vi "Dashboard Main.vi"() -> ()   [LabVIEW 2019]
uses:
  <vilib>/Utility/miscctls.llb/LVRectTypeDef.ctl
  <vilib>/Utility/miscctls.llb/LVRowAndColumnTypeDef.ctl
  <vilib>/event_ctls.llb/eventvkey.ctl
  <vilib>/Rock Robotics/WPI/DriverStation/WPI_DriverStationAllianceInfo.ctl
  <vilib>/Utility/xml.llb/Read From XML File(array).vi
  <vilib>/Utility/xml.llb/Write to XML File(string).vi
  <vilib>/Rock Robotics/Network Tables/NT Write Boolean.vi
  <vilib>/Rock Robotics/Network Tables/NT Read Boolean.vi
  <vilib>/Rock Robotics/Network Tables/NT Read Boolean Array.vi
  <vilib>/Rock Robotics/Network Tables/NT Write Boolean Array.vi
  <vilib>/Rock Robotics/WPI/Dashboard/WPI_DashboardLogging Global.vi
  <vilib>/vision/NI_Vision_Development_Module.lvlib
panel:
  out "Shifter_Faults_Array":bool[](array[boolean])
  out "Drive_Overheat_Array":bool[](array[boolean])
  out "Audible_Warnings_Enabled":bool
  in  "TCP":refnum<k5>
  in  "Rec Mode":enum32{"Stop", "Record", "Playback"}(radio)
  out "Image Message":string="Timeout in Camera Communications"
  in  "Dashboard Tab":T1(tab)=enum."Setup/Auto"
  in  "CheckList":i32(listbox)
  out "Match_End":bool
  out "Auto Playbook Entry":string
  out "Drive Action":string
  out "Subsystem Action":string
  in  "Driver Profile":u16(ring) items=["N/A"]
  in  "Camera Name":string(combo)="limelight"
  in  "Camera Settings":T2={"Frame Rate"=20, "Compression"=60, "Size"=1, "DB Camera Config"=FALSE} {"Size" items=["640x480", "320x240", "160x120"]}
  in  "Autonomous Play":u16(ring) items=["N/A"]
  out "Robot Pose":cluster{dbl[], dbl[]}[](graph)
  out "Master_Caution_0":bool caption="Mode_Butterfly"
  out "Robot_is_Autonomous_0":bool caption="Mode_Butterfly"
  in  "Robot Profile":u16(ring) items=["N/A"]
  out "Robot_Code_Version":string
  in  "Hide_Popups":bool
  in  "Default Camera Pipeline":u16(ring) items=["N/A"]
  in  "Dock_Dashboard":bool
  out "Auto_Suffix":string
  in  "Refresh_Auto_Play_List":bool
  in  "Force_Human_Control":bool
  in  "Auto_Test_Mode":bool
  in  "Auto_Delay":dbl format="%.1f"
  in  "Warning Time (s)":dbl=30.0 format="%.1f"
  in  "Manual_Start_X":dbl=509.25 format="%.1f"
  in  "Disable_Fusion_X":bool=TRUE
  out "Robot X":dbl format="%.1f"
  out "Robot Y":dbl format="%.1f"
  in  "Manual_Start_Y":dbl=94.66 format="%.1f"
  in  "Disable_Fusion_Y":bool=TRUE
  out "Robot H":dbl format="%.1f"
  in  "Manual_Start_H":dbl format="%.1f"
  out "Turret_H":dbl format="%.1f"
  out "Distance_To_Target_Detail":dbl format="%.1f"
  in  "Field Map":u16(ring) items=["N/A"]
  in  "Push_Robot_Start":bool
  in  "Export_Robot_Pose":bool
  in  "Clear_Robot_Pose_Display":bool
  in  "Driver_Help":bool
  in  "Error_Help":bool
  out "Help Graphic":T3(plugin-control)
  out "Drive_Train_Azimuth_Sensor":bool
  out "Camera_Fault":bool
  out "Robot Pose 1":cluster{dbl[], dbl[]}[](graph)
  out "Drive_Train_Shifter":bool
  out "Electrical_Fault":bool
  out "Diverting_Power":bool
  in  "Master_Safety_Override_1":bool
  out "Cowl_A":bool
  out "Cowl_B":bool
  out "Cowl_C":bool
  out "Shooter_Power":dbl(knob) scale=0.0..1.0
  out "Kicker_Power":dbl(knob) scale=0.0..1.0
  out "CAN_Bus_Fault":bool
  out "IMU_Failure":bool
  out "Robot_is_Autonomous_1":bool caption="Mode_Butterfly"
  in  "Pre_Spin":bool
  out "LL_Valid":bool caption="Mode_Butterfly"
  in  "Clear_Jams":bool
  out "Balls_Shot":i32 format="%#.0f"
  out "Ret_Feeder_Left":bool
  out "Ret_Feeder_Right":bool
  out "Climber_Climbing":bool caption="Mode_Butterfly"
  out "Tablet_Override":bool
  out "Match Time(s)":sgl format="%#.0f"
  out "Turret_Azimuth_Failure":bool
  out "Intake_Overheat":bool
  out "Flapper_Flapping":bool caption="Mode_Butterfly"
  out "Ret_Ball_Left":bool
  out "Ret_Ball_Right":bool
  in  "Emergency_Cowl_Retract":bool
  out "Shooter_Motor_Failure":bool
  out "Intake_On":bool caption="Mode_Butterfly"
  out "Shooter_Overheat":bool
  out "Ready_To_Shoot":bool caption="Mode_Butterfly"
  out "Auto_Error":bool
  in  "Clear_Errors":bool
  out "Drive_Train_Azimuth":bool
  out "Pressure_Transducer":dbl(slide) scale=0.0..120.0
  out "Pressure_Leak":bool
  out "Shooter_RPM_Actual":dbl(slide) scale=0.0..5700.0
  out "Drive_Train_Overheat":bool
  out "Compressor_On":bool
  out "Ret_Power_Port_Right":bool
  out "Ret_Power_Port_Left":bool
  in  "Right":bool
  in  "Reticule":T4(ring)
  in  "Save":bool
  in  "Up":bool
  in  "Down":bool
  in  "Left":bool
  out "Master_Caution_1":bool caption="Mode_Butterfly"
  out "Battery_Critical":bool
  out "Battery_Voltage":dbl(slide) scale=11.0..13.0
  out "Field_Oriented":bool caption="Mode_Butterfly"
  in  "Master_Safety_Override_2":bool
  out "Shooter_RPM_Goal":dbl(slide) scale=0.0..5700.0
  out "Slow_Loop":bool
  in  "Mode_TargetingComputer":bool
  in  "Mode_Wall":bool
  in  "Arm_Climber":bool
  in  "State_Normal":bool
  in  "State_Rotation_Control":bool
  in  "State_Climb":bool
  in  "Mode_InitiationLine":bool
  in  "Mode_CloseTrench":bool
  in  "Mode_FarTrench":bool
  in  "State_Position_Control":bool
  out "Combined Camera Feed":T3(plugin-control)
  out "High_Gear_0":bool
  out "High_Gear_1":bool
  out "High_Gear_2":bool
  out "High_Gear_3":bool
  in  "Camera_Override":bool
  out "Shooter_1_Temp":dbl
  out "Shooter_RPM_Goal_Detail":dbl
  out "Wheel_3S_Velocity":dbl format="%.1f"
  out "Wheel_3_Azimuth":dbl format="%.1f"
  out "Wheel_3S_Temp":dbl
  out "Wheel_0S_Temp":dbl
  in  "Select Auto":string(combo)="Select Autonomous ..."
  out "Camera Perf":string
  out "Control Loop Time (ms)":u32
  in  "Super_Test_Mode":bool
  in  "Calibrate_Wheels":bool
  in  "Zero_Wheels":bool
  out "Wheel_0_Azimuth":dbl format="%.1f"
  out "Wheel_0S_Velocity":dbl format="%.1f"
  out "Wheel_1S_Velocity":dbl format="%.1f"
  out "Wheel_1_Azimuth":dbl format="%.1f"
  out "Wheel_1S_Temp":dbl
  out "Wheel_2S_Velocity":dbl format="%.1f"
  out "Wheel_2_Azimuth":dbl format="%.1f"
  out "Wheel_2S_Temp":dbl
  in  "Arm_Calibrate":bool
  out "Shooter_0_RPM_Actual_Detail":dbl
  out "Master_Caution_2":bool caption="Mode_Butterfly"
  out "Shooter_0_Temp":dbl
  out "Shooter_1_RPM_Actual_Detail":dbl
  out "Out_Of_Range":bool
  in  "Wall_Speed":dbl=3000.0 min=0.0 max=5700.0 step=100.0
  in  "Initiation_Line":dbl=2250.0 min=0.0 max=5700.0 step=100.0
  in  "Close_Trench_Speed":dbl=2075.0 min=0.0 max=5700.0 step=100.0
  in  "Far_Trench_Speed":dbl=1975.0 min=0.0 max=5700.0 step=100.0
  out "Kicker_RPM_Actual_Detail":dbl
  out "Kicker_RPM_Goal_Detail":dbl
  out "Kicker_Temp":dbl
  in  "All_Kicker_Speed":dbl=4000.0 min=0.0 max=5700.0 step=100.0
  out "Intake_Temp":dbl
  out "Turret_Azimuth":dbl format="%.1f"
  in  "Arm_Calibrate_Turret":bool
  in  "Calibrate_Turret":bool
  in  "Turret_Override":bool
  in  "Actuator Testing":u16(ring) items=["N/A"]
  in  "Test_Actuator_Value":dbl step=0.1 format="%.2f"
  in  "Zero_Turret":bool
  in  "Auto_Target_Override":bool
  out "Turret_Limit_Switch_A":bool
  out "Turret_Limit_Switch_B":bool
  in  "Calibrate_Joysticks":bool
  in  "Arm_Calibrate_Joysticks":bool
  out "Robot_is_Autonomous_2":bool caption="Mode_Butterfly"
  in  "Test_Actuator_Period":dbl min=0.0 step=1.0 format="%.2f"
  out "Pose Loop Time (ms)":u32
  in  "Mute_Audible_Warnings":bool
  out "Combined Error String":string
  out "LIDAR_Distance_To_Target":dbl format="%.1f"
  out "Beam_Break_Raw":i32
  out "Wheel_0_Shifter_State":string
  out "Wheel_1_Shifter_State":string
  out "Wheel_3_Shifter_State":string
  out "Wheel_2_Shifter_State":string
  out "Azimuth_Error_Array":bool[](array[boolean])
  out "NT Connection":bool
  out "Mode":T5(ring)=enum."Auto Disabled"
  in  "Test Slider":dbl(slide) scale=0.0..100.0 scale format="%#_3g"
  in  "On/Off":bool caption="Solenoid"
  in  "Test Name":u16(ring) items=["Select the test to run..."]
  in  "Test Tree":string(tree)
  in  "Motor":cluster{"Value":dbl, "Enable":bool} {"Value" scale=-1.0..1.0 scale format="%#_3g"}
  out "Progress":T6 {"Test Progress" scale=0.0..100.0}
  in  "Rev/Fwd":cluster{"Forward":bool, "Reverse":bool}
  in  "Test Ring":u16(ring) items=["Monochrome", "Color"]
  out "Cmd Status":string
  in  "Execute Command":bool
  in  "Command Params":string[][](table)
  in  "Command Selection":i32(listbox)
  out "Tree":string(tree)
  out "Background":bool
  # "2020 Dashboard v3.5-stable"
  # "Auto Delay (s)"
  # "Auto Play Suffix"
  # "Robot X (in)"
  # "Endgame Alert (s)"
  # "Robot Y (in)"
  # "Robot H (deg)"
  # "Turret H (deg)"
  # "Undock Dashboard"
  # "Hide\nPopups"
  # "Auto Test\nMode"
  # "Force\nHuman"
  # "Distance (in)"
  # "Drive Action"
  # "Dock Dashboard"
  # "Dynamic Popups"
  # "Auto Real Mode"
  # "Robot\nDecides"
  # "Subsystem Action"
  # "11V"
  # "13V"
  # "0psi"
  # "120psi"
  # "High Gears"
  # "Shooter & Kicker"
  # "Miscellaneous"
  # "Drive Train"
  # "Calibrate Joysticks"
  # "Control"
  # "Pose"
  # "LIDAR\nDistance (in)"
  # "Latency\n(ms)"
  # "Intake"
  # "Module 1"
  # "Module 0"
  # "Shooter"
  # "Kicker"
  # "Azimuth (deg)"
  # "Temp (C)"
  # "Speed Goal (rpm)"
  # "Temp (C)"
  # "Beam Break"
  # "Turret \nOverride"
  # "Auto Target Override"
  # "Camera Override"
  # "Super Test Mode"
  # "Shoot 0"
  # "Shoot 1"
  # "Kicker"
  # "Turret"
  # "Velocity (ft/s)"
  # "Speed (rpm)"
  # "Azimuth (deg)"
  # "Shifter State"
  # "Temp (C)"
  # "Limits"
  # "Module 2"
  # "Module 3"
  # "Setpoints (not saved)"
  # "Azimuth (deg)"
  # "Normal\nTurret"
  # "Normal \nAuto Target"
  # "Normal Camera"
  # "Safe"
  # "Close \nWall"
  # "Initiation\nLine"
  # "Close\nTrench"
  # "Mid\nTrench"
  # "All \nKicker"
  # "Calibrate Turret"
  # "Temp (C)"
  # "Velocity (ft/s)"
  # "(rpm)"
  # "Shifter State"
  # "p: power [-1,1]\nb: boolean {0,1}\nRPM: speed\na: angle [0,+inf)"
  # "Amplitude"
  # "Calibrate Wheels"
  # "Period (s)"
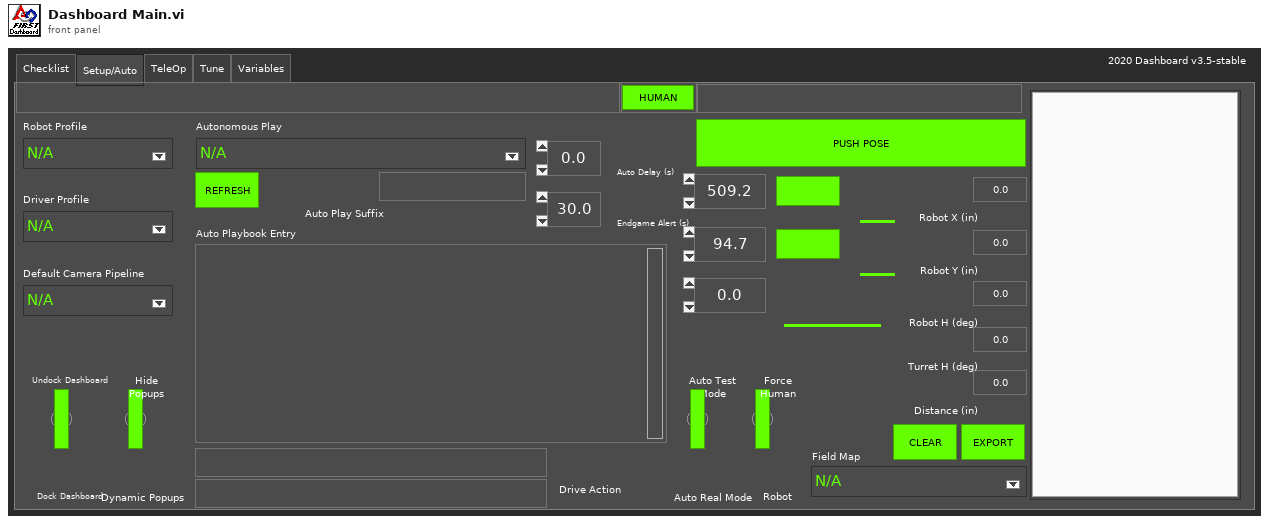
[diagram p1: front panel]
types:
  T1 = enum32{"Checklist", "Setup/Auto", "TeleOp", "Tune", "NT", "Test", "Commands", "Variables"}
  T2 = cluster{"Frame Rate":i32, "Compression":i32, "Size":u16, "DB Camera Config":bool}
  T3 = typedef "IMAQ Image.ctl" = refnum<image>
  T4 = enum16{"Power Port Left", "Power Port Right", "Ball Left", "Ball Right", "Feeder Left", "Feeder Right"}
  T5 = enum8{"Tele-Op Disabled", "Tele-Op Enabled", "Auto Disabled", "Auto Enabled", "Test Disabled", "Test Enabled", "Disconnected", "No Code", "E-Stop"}
  T6 = cluster{"Test Progress":u8, "Test Progress Text":string}
  T7 = cluster{"Save Path":path, "Interval (s)":dbl, "Keep":i32}
  T8 = enum32{"Drive", "Camera", "Basic", "Custom", "Test", "Commands", "Checklist", "Variables"}
  T9 = cluster{"IDs":cluster{"RPC field ID":u16, "Unique ID":u16}, "String":string}
  T10 = typedef "Image Type" = u32
  T11 = cluster{"Ret_Power_Port_Left":refnum<vi>, "Ret_Power_Port_Right":refnum<vi>, "Ret_Ball_Left":refnum<vi>, "Ret_Ball_Right":refnum<vi>, "Ret_Feeder_Left":refnum<vi>, "Ret_Feeder_Right":refnum<vi>}
  T12 = cluster{"Camera Name":string, string, "Saved DB Images Info":cluster{"Save Path":path, "Interval (s)":dbl, "Keep":i32}}
  T13 = enum8{"Enabled", "Disabled", "Disabled and Grayed Out"}
  T14 = typedef "WPI_DriverStationAllianceInfo.ctl" = enum16{"Red", "Blue", "Invalid"}
  T15 = cluster{"Error Strings":string, "Disable Counts":cluster{u16, u16}, "Rail Faults":cluster{u16, u16, u16}, "Robot IP":string, "DB Mode":u8, "Event Info":cluster{"Name":string, "Type":u8, "Number":u16, "Replay":u8}}
  T16 = cluster{"Storage":cluster{"Disk Free":u64, "RAM Block":u32, "RAM free":u32}, "CPU Utilization":cluster{"CPU % ISR":sgl, "CPU % Time Crit":sgl, "CPU % Timed Str":sgl, "CPU % High":sgl, "CPU % Above":sgl, "CPU % Normal":sgl, "CPU % Low":sgl}, "CAN":cluster{"% Bus Utilization":sgl, "Bus Off Cnt":u32, "TX_FIFO Full Cnt":u32, "Receive Error Cnt":u8, "Transmit Error Cnt":u8}, "HID":cluster{"HID Outputs":u32, "Rumble Low":u16, "Rumble High":u16}[]}
  T17 = cluster{"Status bits":cluster{"Test Mode":bool, "Autonomous":bool, "Enabled":bool, "Code Start":bool, "Brownout":bool, "Reserved 2":bool, "Reserved 3":bool, "E-Stop":bool}, "Code Trace":cluster{"Disabled":bool, "TeleOp":bool, "Auto":bool, "Test":bool}, "Controller Type":enum16{"unknown", "cRIO", "roboRio"}, "Code?":enum16{"unknown", "noCode", "code"}, "Battery V":dbl}
  T18 = cluster{"Control Bits":cluster{"TestMode":bool, "Autonomous":bool, "Enabled":bool, "FMS Present":bool, bool, bool, bool, "E-Stop":bool}, "Team Station ":u8, "Countdown":sgl, "Joystick Values":cluster{"Axes":dbl[], "Buttons":bool[], "POVs":i16[]}[]}
  T19 = typedef "imagedata.ctl" = cluster{"image type":i32, "image depth":i32, "image":u8[], "mask":u8[], "colors":u32[], "Rectangle":cluster{"left":i16, "top":i16, "right":i16, "bottom":i16}}
  T20 = cluster{bool, "Super_Test_Mode":bool, "Slow_Loop":bool, "Drive_Train_Overheat":bool, "Pressure_Leak":bool, "Drive_Train_Azimuth":bool, "Arm_Calibrate":bool, "Auto_Error":bool, "Auto_Test_Mode":bool, "Shooter_Overheat":bool, "Shooter_Motor_Failure":bool, "Intake_Overheat":bool, "Turret_Azimuth_Failure":bool, "Arm_Calibrate_Turret":bool, bool, "IMU_Failure":bool, "Electrical_Fault":bool, "Arm_Calibrate_Joysticks":bool, "CAN_Bus_Fault":bool, "Drive_Train_Shifter":bool, "Drive_Train_Azimuth_Sensor":bool, "Battery_Critical":bool}
  T21 = cluster{"Operation":enum16{"Update", "Clear"}, "Color Box":u32}[]
  T22 = typedef "eventvkey.ctl" = enum16{"ASCII", "Enter", "Return", "Shift", "Ctrl", "Alt", "Cmd", "Opt", "Caps", "NumLock", "Clear", "Break", "Up", "Down", "Left", "Right", "Insert", "Delete", "Home", "End", "PageUp", "PageDown", "Escape", "Help", "Pause", "ScrollLock", "F1", "F2", "F3", "F4", "F5", "F6", "F7", "F8", "F9", "F10", "F11", "F12", "F13", "F14", "F15", "F16", "F17", "F18", "F19", "F20", "F21", "F22", "F23", "F24", "Play", "VolumeUp", "VolumeDown", "Mute", "Two Byte Char"}
  T23 = cluster{"Image Size":bool, "Image Type":bool, "Pixel Value":bool, "ROI Information":bool, "Zoom Factor":bool}
  T24 = cluster{"Operation":enum16{"Update", "Clear"}, "Color Box":u32}
  T25 = typedef "LVRowAndColumnTypeDef.ctl" = cluster{"Row":i32, "Column":i32}
  T26 = cluster{"Shift":bool, "Ctrl":bool, "Alt":bool, "Cmd":bool, "Opt":bool}
  T27 = cluster{string, "Drive_Train_Azimuth_Sensor":bool, dbl}
  T28 = cluster{string, "Drive_Train_Overheat":bool, dbl}
  T29 = cluster{string, "Shooter_Motor_Failure":bool, dbl}
  T30 = cluster{string, "Turret_Azimuth_Failure":bool, dbl}
  T31 = cluster{string, "Arm_Calibrate_Turret":bool, dbl}
  T32 = cluster{string, "Arm_Calibrate_Joysticks":bool, dbl}
  T33 = cluster{string, "Drive_Train_Azimuth_Sensor":bool, dbl}[]
  T34 = typedef "LVRectTypeDef.ctl" = cluster{"Left":i16, "Top":i16, "Right":i16, "Bottom":i16}
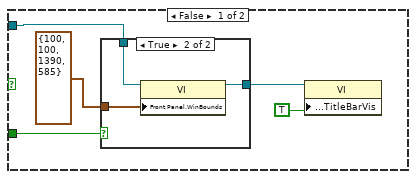
[diagram p2: hidden frame]
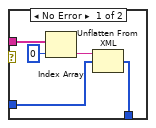
[diagram p6: hidden frame]
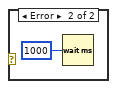
[diagram p9: hidden frame]
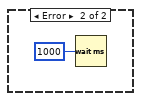
[diagram p10: hidden frame]
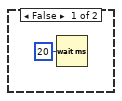
[diagram p11: hidden frame]
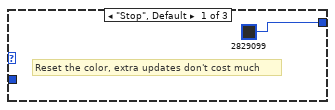
[diagram p15: hidden frame]
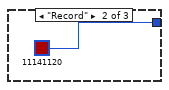
[diagram p16: hidden frame]
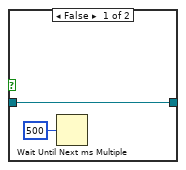
[diagram p19: hidden frame]
diagram:
  w5 = T7 {"Save Path"=path "", "Interval (s)"=1.0, "Keep"=180}  # Saved DB Images Info
  w4 = "Left"
  w16 = T9 {"IDs"={"RPC field ID"=0, "Unique ID"=0}, "String"=""}  # RPC Response
  w26 = enum32{"Stop", "Record", "Playback"}."Stop" ("Rec Mode")
  w20 = FALSE ("Visible")
  w42 = T10 4 items=["Grayscale (U8)", "Grayscale (I16)", "Grayscale (SGL)", "Complex (CSG)", "RGB (U32)", "HSL (U32)", "RGB (U64)"] ("Image Type")
  # "Started one, Unique ID holds\nresponse"
  # "Loop 7. Wait for DS connections"
  # "Basic debug and auto controls: Their data names are fixed, but\nthe displayed name, called a caption, can be changed directly or in\nrobot code such as shown in Begin."
  # "Controls for Test Mode, Camera Settings, etc."
  # "Additional UI Initialization"
  # "Loop 6. Animation for background of window during playback and record"
  # "Fires each time robot IP\nchanges, simulator does this"
  # "Fires each time window\ndocking changes."
  # "The remaining code below this line typically doesn't need to be modified."
  # "Loop 4. Process UI events related to test mode, checklist, and camera settings"
  # "Loop 3. Wait until the robot response provides\n the Robot IP address.\nOnce known, bind controls and\nvariables with the same names."
  n1 = control-ref of="Dashboard Tab"() -> (w24:refnum<vi>)
  n2 = control-ref of="Camera Name"() -> (w11:refnum<vi>)
  n3 = control-ref of="Camera Settings"() -> (w3:refnum<vi>)
  n4 = property class="VI" props=["Front Panel.Closeable"]() -> (reference out=w25:refnum<vi>)  [unwired: 2 in, 2 out]
  n5 = call <vilib>:"Get Tab Control Refs.vi"("Page Index"=T8."Basic" ("Dashboard Tab"), "TabControl in"=w24) -> ("ControlsOnPage"=w10:refnum<vi>[])  [unwired: 9 in]
  n6 = Obtain Notifier(name (unnamed)="Window Mode", notification data type=TRUE) -> (notifier out=w19:refnum<notifier>)  [unwired: 2 in, 2 out]
  n7 = call <vilib>:"Get Tab Control Refs.vi"("Page Index"=T8."Custom" ("Dashboard Tab"), "TabControl in"=w24) -> ("ControlsOnPage"=w23:refnum<vi>[])  [unwired: 9 in]
  n8 = Obtain Notifier(name (unnamed)="Robot IP Update", notification data type="IP Addr" ("name (unnamed)")) -> (notifier out=w2:refnum<notifier>)  [unwired: 2 in, 2 out]
  n9 = Create User Event(user event datatype=w16) -> (user event=w13:refnum<user-event>)  [unwired: 1 in, 1 out]
  n10 = call "IMAQ Create"("Image Name"="Full Video Stream", "Image Type"=w42) -> ("New Image"=w41:T3, "error out"=w40:errorcluster)  [unwired: 2 in, 1 out]
  n11 = Build Array (concatenate)(w10, w23) -> (w22:refnum<vi>[])
  n12 = control-ref of="CheckList"() -> (w21:refnum<vi>)
  n13 = call "Handle Camera Configuration.vi"("CameraNameRef"=w11, "Display Name"=w4, "ClusterRef"=w3) -> ()  [unwired: 9 in]
  n14 = register-events(refnum<vi> refnum, w13) -> (reference out=w30:refnum<event-registration>, error out=w29:errorcluster)  [unwired: 2 in]
  n15 = while {
    tunnel: w22 -> [w54]
    tunnel: w2 -> [w52]
    tunnel: [w50] -> _
    tunnel: u32 1000 ("milliseconds to wait") -> [w49]
    tunnel: w13 -> [w43]
    i -> [w50]
    stop <- FALSE stop-if-true
    n16 = local read "Rec Mode"() -> (w45:enum32{"Stop", "Record", "Playback"})
    n17 = Wait on Notification(notifier=w52, timeout in ms (-1)=w49) -> (notification=w51:string, timed out?=w47:bool)  [unwired: 2 in, 2 out]
    n18 = Equal?(x=w45, y=u16 2 ("Rec Mode")) -> (x = y?=w46:bool)
    n19 = Compound Arithmetic op=OR(invert w47, w46) -> (w48:bool)
    n20 = case shown="True" w48 {
      tunnel: w54 -> [_ w57]
      tunnel: w51 -> [_ w56]
      tunnel: w43 -> [_ w55]
      frame False {
      }
      frame True {
        n21 = call <vilib>:"Bind Controls to SmartDashboard.vi"("RPC ref"=w55, "Bound Control Refs"=w57, "Server IP Address"=w56) -> ()  [unwired: 9 in]
      }
    }
  }
  n22 = while {
    shift-right: [w76] -> _
    shift-left: _ -> [w129]
    shift-right: [w77] -> _
    shift-left: _ -> [w119]
    tunnel: w2 -> [_]
    stop <- FALSE stop-if-true
    # "Dynamic Overlays"
    n23 = To Long Integer(number="Reticule") -> (32bit integer=w110:i32)
    n24 = Wait (ms)(milliseconds to wait=u32 100) -> ()  [unwired: 1 out]
    n25 = Multiply(x=w110, y=2) -> (x*y=w109:i32)
    n26 = control-ref of="Ret_Power_Port_Left"() -> (w90:refnum<vi>)
    n27 = control-ref of="Ret_Power_Port_Right"() -> (w89:refnum<vi>)
    n28 = control-ref of="Ret_Ball_Left"() -> (w75:refnum<vi>)
    n29 = control-ref of="Ret_Ball_Right"() -> (w74:refnum<vi>)
    n30 = control-ref of="Ret_Feeder_Left"() -> (w63:refnum<vi>)
    n31 = control-ref of="Ret_Feeder_Right"() -> (w62:refnum<vi>)
    n32 = Increment(x=w109) -> (x+1=w96:i32)
    n33 = First Call?() -> (First Call?: T/F=w99:bool)
    n34 = Index Array(array=w119, index #1=w109, index #2=w96) -> (element #1=w113:i32, element #2=w121:i32)
    n35 = Or(x="Up", y="Down") -> (x .or. y?=w125:bool)
    n36 = Or(x="Left", y="Right") -> (x .or. y?=w115:bool)
    n37 = case shown="True" w99 {
      tunnel: [w140 w159] -> w76
      tunnel: w129 -> [w140 _]
      tunnel: w90 -> [_ w158]
      tunnel: w89 -> [_ w157]
      tunnel: w75 -> [_ w148]
      tunnel: w74 -> [_ w147]
      tunnel: w63 -> [_ w142]
      tunnel: w62 -> [_ w141]
      frame False {
      }
      frame True {
        n38 = property class="Bool (strict)"(reference=w158) -> ("Left"=w156:i32, "Top"=w155:i32)  [unwired: 1 in, 2 out]
        n39 = property class="Bool (strict)"(reference=w157) -> ("Left"=w154:i32, "Top"=w153:i32)  [unwired: 1 in, 2 out]
        n40 = property class="Bool (strict)"(reference=w148) -> ("Left"=w152:i32, "Top"=w151:i32)  [unwired: 1 in, 2 out]
        n41 = property class="Bool (strict)"(reference=w147) -> ("Left"=w150:i32, "Top"=w149:i32)  [unwired: 1 in, 2 out]
        n42 = property class="Bool (strict)"(reference=w142) -> ("Left"=w146:i32, "Top"=w145:i32)  [unwired: 1 in, 2 out]
        n43 = property class="Bool (strict)"(reference=w141) -> ("Left"=w144:i32, "Top"=w143:i32)  [unwired: 1 in, 2 out]
        n44 = Build Array(w156, w155, w154, w153, w152, w151, w150, w149, w146, w145, w144, w143) -> (w159:i32[])
      }
    }
    n45 = Bundle("Ret_Power_Port_Left"=w90, "Ret_Power_Port_Right"=w89, "Ret_Ball_Left"=w75, "Ret_Ball_Right"=w74, "Ret_Feeder_Left"=w63, "Ret_Feeder_Right"=w62) -> (w81:T11)  [unwired: 1 in]
    n46 = Decrement(x=w121) -> (x-1=w128:i32)
    n47 = Increment(x=w121) -> (x+1=w127:i32)
    n48 = Decrement(x=w113) -> (x-1=w118:i32)
    n49 = Increment(x=w113) -> (x+1=w117:i32)
    n50 = Select(t=w128, s="Up", f=w127) -> (s? t:f=w126:i32)
    n51 = Select(t=w118, s="Left", f=w117) -> (s? t:f=w116:i32)
    n52 = Select(t=w126, s=w125, f=w121) -> (s? t:f=w95:i32)
    n53 = Select(t=w116, s=w115, f=w113) -> (s? t:f=w114:i32)
    n54 = Replace Array Subset(array=w119, new element #1=w114, index #1=w109, new element #2=w95, index #2=w96) -> (w94:i32[])
    n55 = Current VI's Path() -> (path=w105:path)
    n56 = Strip Path(path=w105) -> (stripped path=w104:path)  [unwired: 1 out]
    n57 = Cluster To Array(cluster=w81) -> (array=w93:refnum<vi>[])
    n58 = Strip Path(path=w104) -> (stripped path=w103:path)  [unwired: 1 out]
    n59 = Array Size(array=w93) -> (size(s)=w92:i32)
    n60 = Build Path(base path=w103, name or relative path=path "reticule positions.txt" ("XML File Path")) -> (appended path=w102:path)
    n61 = Multiply(x=2 ("dimension size"), y=w92) -> (x*y=w98:i32)
    n62 = Initialize Array(0, w98) -> (w88:i32[])
    n63 = call-poly <vilib>:"Read From XML File.vi"("XML File Path"=w102) -> ("error out"=w80:errorcluster, "XML Elements"=w101:string[])  [unwired: 8 in, 1 out]
    n64 = case shown="Error .." w80 {
      tunnel: w101 -> [w136 _]
      tunnel: w88 -> [w133 _]
      tunnel: [w132 i32[] [0, 0, 0, 0, 0, 0, 0, 0, 0, 0, 0, 0] ("value")] -> w78
      frame No Error {
        n65 = Index Array(array=w136, index=0) -> (element=w134:string)
        n66 = Unflatten From XML(xml string=w134, type=w133) -> (value=w132:i32[])  [unwired: 1 in, 1 out]
      }
      frame Error {
      }
    }
    n67 = First Call?() -> (First Call?: T/F=w120:bool)
    n68 = Select(t=w78, s=w120, f=w94) -> (s? t:f=w77:i32[])
    n69 = Add(x=w77, y=w76) -> (x+y=w79:i32[])
    n70 = Index Array(array=w79, index #1=0 ("index")) -> (element #1=w85:i32, element #2=w84:i32, element #3=w83:i32, element #4=w82:i32, element #5=w73:i32, element #6=w72:i32, element #7=w71:i32, element #8=w70:i32, element #9=w67:i32, element #10=w66:i32, element #11=w65:i32, element #12=w64:i32)  [unwired: 11 in]
    n71 = Unbundle(w81) -> ("Ret_Power_Port_Left"=w86:refnum<vi>, "Ret_Power_Port_Right"=w87:refnum<vi>, "Ret_Ball_Left"=w69:refnum<vi>, "Ret_Ball_Right"=w68:refnum<vi>, "Ret_Feeder_Left"=w61:refnum<vi>, "Ret_Feeder_Right"=w60:refnum<vi>)
    n72 = Flatten To XML(anything=w77) -> (xml string=w107:string)
    n73 = call "EdgeTrigger.vi"("Input Signal"="Save") -> ("Rising Edge Trigger"=w58:bool)  [unwired: 2 out]
    n74 = case shown="True" w58 {
      tunnel: w107 -> [_ w139]
      tunnel: w102 -> [_ w138]
      frame False {
      }
      frame True {
        n75 = call-poly <vilib>:"Write to XML File.vi"("XML Input"=w139, "XML File Path"=w138) -> ()  [unwired: 7 in, 3 out]
      }
    }
    n76 = property class="Bool (strict)"(reference=w86, "Left"=w85, "Top"=w84) -> ()  [unwired: 1 in, 2 out]
    n77 = property class="Bool (strict)"(reference=w87, "Left"=w83, "Top"=w82) -> ()  [unwired: 1 in, 2 out]
    n78 = property class="Bool (strict)"(reference=w69, "Left"=w73, "Top"=w72) -> ()  [unwired: 1 in, 2 out]
    n79 = property class="Bool (strict)"(reference=w68, "Left"=w71, "Top"=w70) -> ()  [unwired: 1 in, 2 out]
    n80 = property class="Bool (strict)"(reference=w61, "Left"=w67, "Top"=w66) -> ()  [unwired: 1 in, 2 out]
    n81 = property class="Bool (strict)"(reference=w60, "Left"=w65, "Top"=w64) -> ()  [unwired: 1 in, 2 out]
  }
  n82 = while {
    tunnel: w41 -> [w175]
    tunnel: w40 -> [_]
    tunnel: w5 -> [w180]
    tunnel: w4 -> [w178]
    stop <- FALSE stop-if-true
    # "Camera Feeds"
    n83 = local read "NT Connection"() -> (w181:bool)
    n84 = local read "Rec Mode"() -> (w182:enum32{"Stop", "Record", "Playback"})
    n85 = Bundle("Camera Name"="Camera Name", w178, "Saved DB Images Info"=w180) -> (w179:T12)  [unwired: 1 in]
    n86 = control-ref of="Camera Perf"() -> (w176:refnum<vi>)
    n87 = call <vilib>:"WPI_CameraRead MJPG for Dashboard_2.vi"("Camera Settings"="Camera Settings", "Rec Mode"=w182, "NT Connection"=w181, "Capture Info"=w179, "Image in"=w175) -> ("perf info"=w177:cluster{"Bandwidth (Mbps)":dbl, "fps":dbl}, "Active"=w183:bool, "Image\\ out"=w184:T3)  [unwired: 4 in]
    n88 = call <vilib>:"WPI_DashboardFormatPerf.vi"("Right Camera Perf"=cluster{"Bandwidth (Mbps)":dbl, "FPS":dbl} {"Bandwidth (Mbps)"=0.0, "FPS"=0.0}, "Performance"=w177, "String in"=w176) -> ()  [unwired: 9 in]
    n89 = case shown="True" w183 {
      tunnel: w184 -> [w197 w200]
      tunnel: [w197 w199] -> w174
      frame False {
        n90 = Wait Until Next ms Multiple(millisecond multiple=u32 500) -> ()  [unwired: 1 out]
      }
      frame True {
        # "image annotation etc."
        n91 = call "IMAQ Clear Overlay"("Image"=w200) -> ("Image Out"=w199:T3)  [unwired: 2 in, 8 out]
      }
    }
    n92 = call "IMAQ Rotate"("Angle (degrees)"=sgl 0.0, "Image Src"=w174) -> ("Image Dst Out"=w163:T3)  [unwired: 8 in, 1 out]
    n93 = call "IMAQ GetImageSize"("Image"=w163) -> ("Y Resolution"=w169:i32, "X Resolution"=w170:i32)  [unwired: 3 in, 1 out]
    n94 = To Double Precision Float(number=w170) -> (double precision float=w172:dbl)
    n95 = To Double Precision Float(number=w169) -> (double precision float=w171:dbl)
    n96 = Divide(x=w172, y=w171) -> (x/y=w168:dbl)
    n97 = Less?(x=w168, y=1.5) -> (x < y?=w160:bool)
    "Camera_Fault" <- w160
    n98 = case shown="True" w160 {
      tunnel: "Partial Video Stream" ("Image Name") -> [_ w196]
      tunnel: [w186 w195] -> w162
      tunnel: w163 -> [w186 w191]
      frame False {
        # "wide angle camera found"
      }
      frame True {
        # "no wide angle camera found"
        n99 = call "IMAQ GetImageInfo"("Image"=w191) -> ("Y Resolution"=w190:i32, "X Resolution"=w189:i32, "Image Type"=w194:T10)  [unwired: 3 in, 5 out]
        n100 = call "IMAQ Create"("Image Name"=w196, "Image Type"=w194) -> ("New Image"=w193:T3)  [unwired: 3 in, 1 out]
        n101 = Multiply(x=w189, y=2) -> (x*y=w188:i32)
        n102 = call "IMAQ SetImageSize"("Y Resolution"=w190, "X Resolution"=w188, "Image"=w193) -> ("Image Out"=w192:T3)  [unwired: 2 in, 1 out]
        n103 = call "IMAQ ImageToImage 2"("Image Src (Small)"=w191, "Image Src (Large)"=w192) -> ("Image Dst Out"=w195:T3)  [unwired: 8 in, 1 out]
      }
    }
    "Combined Camera Feed" <- w162
  }
  n104 = call "Initialize Camera and CheckList.vi"("ListBox in"=w21) -> ()  [unwired: 11 in]
  n105 = control-ref of="Test Tree"() -> (w35:refnum<vi>)
  n106 = while {
    tunnel: w2 -> [w204]
    tunnel: w19 -> [w201]
    stop <- FALSE stop-if-true
    n107 = call <vilib>:"WPI_DashboardRetrieveStatusInfo.vi"("Binding Refnum"=w204, "Window Mode Notifier"=w201, "TCP Cnx"="TCP") -> ("Power and Errors"=w205:T15, "Robot Metrics"=w208:T16, "Status Info"=w209:T17, "Control Info"=w206:T18, "Robot Mode"=w203:T5, "Process?"=w207:bool)  [unwired: 3 in]
    "Mode" <- w203
    n108 = case shown="True" w207 {
      tunnel: w209 -> [_ _]
      tunnel: w208 -> [_ _]
      tunnel: w206 -> [_ _]
      tunnel: w205 -> [_ _]
      tunnel: w203 -> [_ _]
      frame False {
        n109 = Wait (ms)(milliseconds to wait=u32 20) -> ()  [unwired: 1 out]
      }
      frame True {
        w216 = "H" ("x")
        w222 = bool[] [FALSE, FALSE, FALSE, FALSE] ("Default Value")
        w269 = FALSE  # Compressor
        w264 = FALSE
        w272 = FALSE  # LimeLight
        w595 = cluster{u32, u32}[] [{15663313, 16448250}, {16448250, 16448250}] ("Un-selected Color")
        w541 = cluster{u32, u32}[] [{9567230, 16448250}, {16448250, 16448250}] ("Un-selected Color")
        # "# of false elements"
        # "Find # of trues"
        # "manage audible warnings"
        # "robot configuration"
        # "manipulator controls"
        # "spinner reporting"
        # "report targeting information"
        # "report tab position"
        # "tuning parameters and calibrations"
        # "climber reporting"
        # "turret reporting"
        # "intake and magazine reporting"
        # "drive system reporting"
        # "report resource usage"
        # "dynamic overlays"
        # "shooter reporting"
        # "shooter state controller"
        # "master state controller"
        # "report match time"
        # "actuator test interlocks"
        # "emergency overrides"
        # "caution alarms"
        # "driver configuration"
        # "autonomous reporting"
        # "autonomous configuration"
        # "display auto \nplaybook"
        n110 = call-poly <vilib>:"NT Read Value.vi"("Name"="Alliance_Color") -> ("Numeric"=w702:dbl)  [unwired: 9 in, 1 out]
        n111 = To Unsigned Word Integer(number=w702) -> (unsigned 16bit integer=w701:u16)
        n112 = call-poly <vilib>:"NT Read Value.vi"("Name"="Robot_Mode") -> ("String"=w343:string)  [unwired: 9 in, 1 out]
        n113 = Build Array("N/A") -> (w791:string[])
        n114 = call-poly <vilib>:"NT Read Value.vi"("Default Value"=0.0, "Name"="Robot_H") -> ("Numeric"=w351:dbl)  [unwired: 8 in, 1 out]
        n115 = call-poly <vilib>:"NT Read Value.vi"("Default Value"=0.0, "Name"="Turret_H") -> ("Numeric"=w350:dbl)  [unwired: 8 in, 1 out]
        n116 = feedback-in #1(w701) -> ()
        n117 = feedback #1(w701) -> (w709:u16)
        n118 = Not Equal?(x=w701, y=w709) -> (x != y?=w707:bool)
        n119 = feedback #2("Field Map") -> (w301:u16)
        n120 = feedback-in #2("Field Map") -> ()
        n121 = Not Equal?(x="Field Map", y=w301) -> (x != y?=w299:bool)
        n122 = call-poly <vilib>:"NT Read Value.vi"("Default Value"=-1.0, "Name"="Robot_Y") -> ("Numeric"=w353:dbl)  [unwired: 8 in, 1 out]
        "Robot Y" <- w353
        n123 = call-poly <vilib>:"NT Read Value.vi"("Default Value"=-1.0, "Name"="Robot_X") -> ("Numeric"=w354:dbl)  [unwired: 8 in, 1 out]
        "Robot X" <- w354
        n124 = First Call?() -> (First Call?: T/F=w708:bool)
        n125 = call-poly <vilib>:"NT Read Value.vi"("Default Value"=w791, "Name"="Legal_Auto_Plays") -> ("String Array"=w789:string[])  [unwired: 8 in, 1 out]
        n126 = To Double Precision Float(number="Autonomous Play") -> (double precision float=w795:dbl)
        n127 = call-poly <vilib>:"NT Read Value.vi"("Default Value"="Waiting for connection...", "Name"="Auto_Playbook") -> ("String"=→"Auto Playbook Entry":string)  [unwired: 8 in, 1 out]
        n128 = Quotient & Remainder(x=w351, y=360.0) -> (x-y*floor(x/y)=→"Robot H":dbl)  [unwired: 1 out]
        n129 = Quotient & Remainder(x=w350, y=360.0) -> (x-y*floor(x/y)=→"Turret_H":dbl)  [unwired: 1 out]
        n130 = call-poly <vilib>:"NT Read Value.vi"("Name"="Auto_Path_Suffix") -> ("String"=→"Auto_Suffix":string)  [unwired: 9 in, 1 out]
        n131 = Compound Arithmetic op=OR(w707, w708, w299) -> (w706:bool)
        n132 = call-poly <vilib>:"NT Write Value.vi"("Boolean"="Disable_Fusion_X", "Name"="Disable_Fusion_X") -> ()  [unwired: 9 in, 1 out]
        n133 = call-poly <vilib>:"NT Write Value.vi"("Boolean"="Disable_Fusion_Y", "Name"="Disable_Fusion_Y") -> ()  [unwired: 9 in, 1 out]
        n134 = call-poly <vilib>:"NT Write Value.vi"("Boolean"="Push_Robot_Start", "Name"="Push_Robot_Start") -> ()  [unwired: 9 in, 1 out]
        n135 = call-poly <vilib>:"NT Write Value.vi"("Boolean"="Auto_Test_Mode", "Name"="Auto_Test_Mode") -> ()  [unwired: 9 in, 1 out]
        n136 = call-poly <vilib>:"NT Write Value.vi"("Numeric"="Auto_Delay", "Name"="Auto_Delay") -> ()  [unwired: 9 in, 1 out]
        n137 = call-poly <vilib>:"NT Write Value.vi"("Numeric"="Manual_Start_X", "Name"="Manual_Start_X") -> ()  [unwired: 9 in, 1 out]
        n138 = call-poly <vilib>:"NT Write Value.vi"("Numeric"="Manual_Start_Y", "Name"="Manual_Start_Y") -> ()  [unwired: 9 in, 1 out]
        n139 = call-poly <vilib>:"NT Write Value.vi"("Numeric"="Manual_Start_H", "Name"="Manual_Start_H") -> ()  [unwired: 9 in, 1 out]
        n140 = call-poly <vilib>:"NT Write Value.vi"("Boolean"="Force_Human_Control", "Name"="Force_Human_Control") -> ()  [unwired: 9 in, 1 out]
        n141 = call-poly <vilib>:"NT Write Value.vi"("Boolean"="Refresh_Auto_Play_List", "Name"="Refresh_Auto_Play_List") -> ()  [unwired: 9 in, 1 out]
        n142 = call-poly <vilib>:"NT Write Value.vi"("Numeric"=w795, "Name"="Selected_Auto_Play") -> ()  [unwired: 9 in, 1 out]
        n143 = case shown="True" w706 {
          tunnel: w701 -> [_ w847]
          tunnel: "Field Map" -> [_ w845]
          frame False {
          }
          frame True {
            # "load and field map"
            n144 = To Long Integer(number=w845) -> (32bit integer=w843:i32)
            n145 = Current VI's Path() -> (path=w850:path)
            n146 = Strip Path(path=w850) -> (stripped path=w849:path)  [unwired: 1 out]
            n147 = Strip Path(path=w849) -> (stripped path=w846:path)  [unwired: 1 out]
            n148 = List Folder(path=w846, pattern="*map*.png") -> (filenames=w844:string[])  [unwired: 2 in, 3 out]
            n149 = Index Array(array=w844, index=w843) -> (element=w842:string)
            n150 = property on="Field Map" class="Ring (strict)"("Strings []"=w844) -> ()  [unwired: 2 in, 2 out]
            n151 = Build Path(base path=w846, name or relative path=w842) -> (appended path=w848:path)
            n152 = call <vilib>:"Read PNG File.vi"("path to PNG file"=w848) -> ("error out"=w852:errorcluster, "image data"=w851:T19)  [unwired: 8 in, 1 out]
            n153 = case shown="No Error" w852 {
              tunnel: w851 -> [w870 _]
              tunnel: w847 -> [w854 _]
              frame No Error {
                w871 = T10 4 items=["Grayscale (U8)", "Grayscale (I16)", "Grayscale (SGL)", "Complex (CSG)", "RGB (U32)", "HSL (U32)", "RGB (U64)", "Grayscale (U16)"] ("Image Type")
                n154 = call <vilib>:"Unflatten Pixmap.vi"("image data"=w870) -> ("24-bit pixmap"=w869:u32[][])  [unwired: 4 in, 6 out]
                n155 = property on="Robot Pose" class="XYGraph (strict)"() -> ("Width"=w874:u32, "Height"=w873:u32)  [unwired: 2 in, 2 out]
                n156 = call "IMAQ Create"("Image Name"="field", "Image Type"=w871) -> ("New Image"=w868:T3)  [unwired: 3 in, 1 out]
                n157 = Equal?(x=w854, y=WPI_DriverStationAllianceInfo."Red" ("x")) -> (x = y?=w856:bool)
                n158 = call "IMAQ ArrayToColorImage"("Image Pixels (U32)"=w869, "Image"=w868) -> ("Image Out"=w867:T3)  [unwired: 3 in, 1 out]
                n159 = To Long Integer(number=w874) -> (32bit integer=w863:i32)
                n160 = To Long Integer(number=w873) -> (32bit integer=w864:i32)
                n161 = call "IMAQ Resample"("X Resolution"=w863, "Y Resolution"=w864, "Image Src"=w867) -> ("Image Dst Out"=w862:T3)  [unwired: 7 in, 1 out]
                n162 = Select(t=180.0, s=w856, f=0.0) -> (s? t:f=w860:dbl)
                n163 = To Single Precision Float(number=w860) -> (single precision float=w859:sgl)
                n164 = call "IMAQ Rotate"("Angle (degrees)"=w859, "Image Src"=w862) -> ("Image Dst Out"=w861:T3)  [unwired: 8 in, 1 out]
                n165 = call "IMAQ ColorImageToArray"("Image"=w861) -> ("Image Pixels (U32)"=w866:u32[][])  [unwired: 3 in, 2 out]
                n166 = call <vilib>:"Flatten Pixmap.vi"("24-bit pixmap"=w866) -> ("image data"=w865:T19)  [unwired: 10 in]
                n167 = call <vilib>:"Draw Flattened Pixmap.vi"("image data"=w865) -> ("new picture"=w853:picture)  [unwired: 8 in]
                n168 = property on="Robot Pose" class="XYGraph (strict)"("PlotImages.Back"=w853) -> ()  [unwired: 2 in, 2 out]
                n169 = property on="Robot Pose 1" class="XYGraph (strict)"("PlotImages.Back"=w853) -> ()  [unwired: 2 in, 2 out]
              }
              frame Error {
              }
            }
          }
        }
        n170 = property on="Autonomous Play" class="Ring (strict)"("Strings []"=w789) -> ()  [unwired: 2 in, 2 out]
        n171 = Equal?(x=w343, y="Teleop Enabled") -> (x = y?=w342:bool)
        n172 = Equal?(x=w343, y="Autonomous Enabled") -> (x = y?=w340:bool)
        n173 = Or(x=w340, y=w342) -> (x .or. y?=w341:bool)
        n174 = call "EdgeTrigger.vi"("Input Signal"=w340) -> ("Rising Edge Trigger"=w304:bool)  [unwired: 2 out]
        n175 = call-poly <vilib>:"NT Read Value.vi"("Name"="Robot_Mode") -> ("String"=w433:string)  [unwired: 9 in, 1 out]
        n176 = Or(x="Clear_Robot_Pose_Display", y=w304) -> (x .or. y?=w303:bool)
        n177 = call "RenderRobotPose.vi"("Robot X (in)"=w354, "Robot Width (in)"=30.5 ("Robot Size (in)"), "Robot Length (in)"=30.5 ("Robot Width (in)"), "Buffer Time (min)"=5.0, "Robot Y (in)"=w353, "Robot Heading (deg)"=w351, "Turret Heading (deg)"=w350, "Robot Enabled"=w341, "Reset"=w303) -> ("Robot Pose"=→"Robot Pose" →"Robot Pose 1":cluster{dbl[], dbl[]}[])  [unwired: 6 in]
        n178 = call-poly <vilib>:"NT Read Value.vi"("Default Value"=0.0, "Name"="Remaining_Time") -> ("Numeric"=w429:dbl)  [unwired: 8 in, 1 out]
        n179 = call "EdgeTrigger.vi"("Input Signal"="Export_Robot_Pose") -> ("Rising Edge Trigger"=w349:bool)  [unwired: 2 out]
        n180 = local read "Robot_is_Autonomous_0"() -> (w308:bool)
        n181 = call-poly <vilib>:"NT Read Value.vi"("Default Value"=13.0, "Name"="Battery_Voltage") -> ("Numeric"=→"Battery_Voltage":dbl)  [unwired: 8 in, 1 out]
        n182 = call-poly <vilib>:"NT Read Value.vi"("Name"="Pose_Loop_Time") -> ("Numeric"=w417:dbl)  [unwired: 9 in, 1 out]
        n183 = call-poly <vilib>:"NT Read Value.vi"("Name"="Control_Loop_Time") -> ("Numeric"=w825:dbl)  [unwired: 9 in, 1 out]
        n184 = call-poly <vilib>:"NT Read Value.vi"("Name"="CAN_Bus_Fault") -> ("Boolean"=→"CAN_Bus_Fault":bool)  [unwired: 9 in, 1 out]
        n185 = case shown="True" w349 {
          frame False {
          }
          frame True {
            # "export the current robot pose data"
            n186 = Get Date/Time In Seconds() -> (seconds since 1Jan1904=w840:timestamp)
            n187 = Format Date/Time String(time format string (%c)="%Y-%m-%d_%H-%M", seconds (now)=w840) -> (date/time string=w838:string)  [unwired: 1 in]
            n188 = Concatenate Strings("robot pose data " ("string"), w838) -> (w836:string)
            n189 = Current VI's Path() -> (path=w835:path)
            n190 = String To Path(string=w836) -> (path=w832:path)
            n191 = Strip Path(path=w835) -> (stripped path=w834:path)  [unwired: 1 out]
            n192 = Strip Path(path=w834) -> (stripped path=w833:path)  [unwired: 1 out]
            n193 = Build Path(base path=w833, name or relative path=w832) -> (appended path=w831:path)
            n194 = invoke on="Robot Pose" class="XYGraph (strict)" method="Export Image"("FileType"=enum32{"BMP", "EPS", "EMF", "PICT"}."BMP" ("File Type"), "Target"=enum32{"File", "Clipboard"}."File", "Path"=w831, "HideGrid"=TRUE ("Hide Grid"), "Overwrite"=TRUE ("Always Overwrite")) -> ()  [unwired: 3 in, 8 out]
          }
        }
        n195 = call-poly <vilib>:"NT Read Value.vi"("Name"="Control_Latency_Alarm") -> ("Boolean"=w444:bool)  [unwired: 9 in, 1 out]
        "Slow_Loop" <- w444
        n196 = call-poly <vilib>:"NT Read Value.vi"("Name"="Battery_Critical") -> ("Boolean"=→"Battery_Critical":bool)  [unwired: 9 in, 1 out]
        n197 = Equal?(x=w433, y="Teleop Enabled") -> (x = y?=w432:bool)
        n198 = call-poly <vilib>:"NT Read Value.vi"("Name"="Electrical_Fault") -> ("Boolean"=→"Electrical_Fault":bool)  [unwired: 9 in, 1 out]
        n199 = call-poly <vilib>:"NT Read Value.vi"("Name"="Diverting_Power") -> ("Boolean"=→"Diverting_Power":bool)  [unwired: 9 in, 1 out]
        n200 = call-poly <vilib>:"NT Read Value.vi"("Name"="Compressor_On") -> ("Boolean"=→"Compressor_On":bool)  [unwired: 9 in, 1 out]
        n201 = call-poly <vilib>:"NT Read Value.vi"("Name"="Pressure_Leak") -> ("Boolean"=→"Pressure_Leak":bool)  [unwired: 9 in, 1 out]
        n202 = call-poly <vilib>:"NT Read Value.vi"("Name"="Pressure_Transducer") -> ("Numeric"=→"Pressure_Transducer":dbl)  [unwired: 9 in, 1 out]
        n203 = call-poly <vilib>:"NT Read Value.vi"("Name"="Robot_is_Autonomous") -> ("Boolean"=→"Robot_is_Autonomous_0" →"Robot_is_Autonomous_1" →"Robot_is_Autonomous_2":bool)  [unwired: 9 in, 1 out]
        n204 = Greater Or Equal To 0?(x=w429) -> (x >= 0?=w428:bool)
        n205 = Less?(x=w429, y="Warning Time (s)") -> (x < y?=w805:bool)
        n206 = call-poly <vilib>:"NT Read Value.vi"("Name"="Auto_Subsytem_Action") -> ("String"=→"Subsystem Action":string)  [unwired: 9 in, 1 out]
        n207 = call-poly <vilib>:"NT Read Value.vi"("Name"="Auto_Drive_Action") -> ("String"=→"Drive Action":string)  [unwired: 9 in, 1 out]
        n208 = call-poly <vilib>:"NT Read Value.vi"("Name"="Auto_Error") -> ("Boolean"=→"Auto_Error":bool)  [unwired: 9 in, 1 out]
        n209 = To Unsigned Long Integer(number=w417) -> (unsigned 32bit integer=→"Pose Loop Time (ms)":u32)
        n210 = To Unsigned Long Integer(number=w825) -> (unsigned 32bit integer=→"Control Loop Time (ms)":u32)
        n211 = Compound Arithmetic op=AND(w428, w805, w432) -> (w467:bool)
        "Match_End" <- w467
        n212 = call "BlinkLight.vi"() -> ("Blinked"=w807:bool)  [unwired: 1 in]
        n213 = Not(x="Hide_Popups") -> (.not. x?=w306:bool)
        n214 = In Range and Coerce(upper limit=inf, x=w429, lower limit=0.0) -> (coerced(x)=w804:dbl)  [unwired: 1 out]
        n215 = Select(t=u32 16711680 ("Numeric Text.Text Colors:Text Color"), s=w444, f=u32 4934475 ("Numeric Text.Text Colors:Text Color")) -> (s? t:f=w682:u32)
        n216 = To Single Precision Float(number=w804) -> (single precision float=→"Match Time(s)":sgl)
        n217 = And(x=w306, y=w308) -> (x .and. y?=w309:bool)
        n218 = Select(t=w807, s=w467, f=FALSE) -> (s? t:f=w778:bool)
        n219 = property on="Control Loop Time (ms)" class="DigNum (strict)"("NumText.BG Color"=w682) -> ()  [unwired: 2 in, 2 out]
        n220 = property on="Robot Pose 1" class="XYGraph (strict)"("Visible"=w309) -> ()  [unwired: 2 in, 2 out]
        n221 = Select(t=u32 16760064 ("Numeric Text.Text Colors:Text Color"), s=w778, f=u32 16448250 ("Numeric Text.Text Colors:Text Color")) -> (s? t:f=w780:u32)
        n222 = local read "Dashboard Tab"() -> (w823:T1)
        n223 = property on="Match Time(s)" class="DigNum (strict)"("NumText.TextColor"=w780) -> ()  [unwired: 2 in, 2 out]
        n224 = Build Array("N/A") -> (w784:string[])
        n225 = And(x="Calibrate_Joysticks", y="Arm_Calibrate_Joysticks") -> (x .and. y?=w437:bool)
        n226 = To Double Precision Float(number="Driver Profile") -> (double precision float=w798:dbl)
        n227 = local read "Drive_Overheat_Array"() -> (w263:bool[])
        n228 = call-poly <vilib>:"NT Read Value.vi"("Name"="LL_Valid") -> ("Boolean"=→"LL_Valid":bool)  [unwired: 9 in, 1 out]
        n229 = call-poly <vilib>:"NT Read Value.vi"("Name"="Distance_To_Target") -> ("Numeric"=→"Distance_To_Target_Detail":dbl)  [unwired: 9 in, 1 out]
        n230 = local read "Azimuth_Error_Array"() -> (w257:bool[])
        n231 = call-poly <vilib>:"NT Read Value.vi"("Default Value"=w784, "Name"="Legal_Drivers") -> ("String Array"=w786:string[])  [unwired: 8 in, 1 out]
        n232 = local read "Shifter_Faults_Array"() -> (w252:bool[])
        n233 = Build Array("N/A") -> (w420:string[])
        n234 = Build Array("N/A") -> (w293:string[])
        n235 = Equal?(x=w823, y=T1."Tune") -> (x = y?=w822:bool)
        n236 = Not(x="Arm_Calibrate_Joysticks") -> (.not. x?=w439:bool)
        n237 = call-poly <vilib>:"NT Write Value.vi"("Numeric"=w798, "Name"="Selected_Driver") -> ()  [unwired: 9 in, 1 out]
        n238 = property on="Driver Profile" class="Ring (strict)"("Strings []"=w786) -> ()  [unwired: 2 in, 2 out]
        n239 = To Double Precision Float(number="Robot Profile") -> (double precision float=w425:dbl)
        n240 = call-poly <vilib>:"NT Write Value.vi"("Boolean"=w822, "Name"="Tune_Tab") -> ()  [unwired: 9 in, 1 out]
        n241 = local read "CAN_Bus_Fault"() -> (w267:bool)
        n242 = local read "Intake_Overheat"() -> (w265:bool)
        n243 = local read "Battery_Critical"() -> (w275:bool)
        n244 = local read "Electrical_Fault"() -> (w274:bool)
        n245 = call-poly <vilib>:"NT Read Value.vi"("Default Value"=w420, "Name"="Legal_Robots") -> ("String Array"=w422:string[])  [unwired: 8 in, 1 out]
        n246 = local read "Pressure_Leak"() -> (w268:bool)
        n247 = call-poly <vilib>:"NT Write Value.vi"("Boolean"=w437, "Name"="Calibrate_Joysticks") -> ()  [unwired: 9 in, 1 out]
        n248 = call-poly <vilib>:"NT Read Value.vi"("Default Value"=w293, "Name"="Legal_Pipelines") -> ("String Array"=w295:string[])  [unwired: 8 in, 1 out]
        n249 = local read "IMU_Failure"() -> (w266:bool)
        n250 = call-poly <vilib>:"NT Write Value.vi"("Numeric"=w425, "Name"="Selected_Robot") -> ()  [unwired: 9 in, 1 out]
        n251 = call-poly <vilib>:"NT Read Value.vi"("Default Value"="No robot code versioning information...", "Name"="Robot_Code_Version") -> ("String"=→"Robot_Code_Version":string)  [unwired: 8 in, 1 out]
        n252 = local read "Slow_Loop"() -> (w273:bool)
        n253 = To Double Precision Float(number="Default Camera Pipeline") -> (double precision float=w298:dbl)
        n254 = property on="Robot Profile" class="Ring (strict)"("Strings []"=w422) -> ()  [unwired: 2 in, 2 out]
        n255 = Select(t=cluster{u32, u32}[] [{11776947, 16448250}, {16448250, 16448250}] ("Colors [4]"), s=w439, f=cluster{u32, u32}[] [{6618880, 16448250}, {16448250, 16448250}] ("Colors [4]")) -> (s? t:f=w438:cluster{u32, u32}[])
        n256 = property on="Default Camera Pipeline" class="Ring (strict)"("Strings []"=w295) -> ()  [unwired: 2 in, 2 out]
        n257 = call-poly <vilib>:"NT Write Value.vi"("Numeric"=w298, "Name"="Selected_Default_Pipeline") -> ()  [unwired: 9 in, 1 out]
        n258 = Index Array(array=w263) -> (element #1=w262:bool, element #2=w261:bool, element #3=w260:bool, element #4=w259:bool)  [unwired: 4 in]
        n259 = Index Array(array=w257) -> (element #1=w258:bool, element #2=w256:bool, element #3=w255:bool, element #4=w254:bool)  [unwired: 4 in]
        n260 = Index Array(array=w252) -> (element #1=w251:bool, element #2=w250:bool, element #3=w249:bool, element #4=w248:bool)  [unwired: 4 in]
        n261 = property on="Calibrate_Joysticks" class="Bool"("Colors [4]"=w438) -> ()  [unwired: 2 in, 2 out]
        n262 = local read "Drive_Train_Azimuth_Sensor"() -> (w279:bool)
        n263 = Build Array(w275, w274, w273, w272, w269, w268, w267, w266, w262, w261, w260, w259, w258, w256, w255, w254, w251, w250, w249, w248, w265) -> (w246:bool[])
        n264 = local read "Master_Safety_Override_1"() -> (w814:bool)
        n265 = local read "Master_Safety_Override_2"() -> (w813:bool)
        n266 = local read "Arm_Calibrate_Joysticks"() -> (w380:bool)
        n267 = local read "Turret_Azimuth_Failure"() -> (w385:bool)
        n268 = local read "Shooter_Motor_Failure"() -> (w387:bool)
        n269 = property on="Actuator Testing" class="Ring (strict)"() -> ("RingText.Text"=w487:string)  [unwired: 2 in, 2 out]
        n270 = local read "Drive_Train_Overheat"() -> (w394:bool)
        n271 = local read "Arm_Calibrate_Turret"() -> (w384:bool)
        n272 = local read "Drive_Train_Azimuth"() -> (w392:bool)
        n273 = local read "Drive_Train_Shifter"() -> (w311:bool)
        n274 = local read "Shooter_Overheat"() -> (w388:bool)
        n275 = local read "Super_Test_Mode"() -> (w396:bool)
        n276 = local read "Auto_Test_Mode"() -> (w389:bool)
        n277 = local read "Intake_Overheat"() -> (w386:bool)
        n278 = local read "Battery_Critical"() -> (w276:bool)
        n279 = local read "CAN_Bus_Fault"() -> (w379:bool)
        n280 = local read "Electrical_Fault"() -> (w381:bool)
        n281 = local read "Compressor_On"() -> (w270:bool)
        n282 = local read "Arm_Calibrate"() -> (w391:bool)
        n283 = local read "Pressure_Leak"() -> (w393:bool)
        n284 = local read "Out_Of_Range"() -> (w459:bool)
        n285 = local read "Camera_Fault"() -> (w271:bool)
        n286 = local read "IMU_Failure"() -> (w382:bool)
        n287 = local read "Slow_Loop"() -> (w395:bool)
        n288 = local read "Auto_Error"() -> (w390:bool)
        n289 = call-poly <vilib>:"NT Read Value.vi"("Name"="Power_Port_Target") -> ("Boolean"=w283:bool)  [unwired: 9 in, 1 out]
        n290 = Not Equal?(x=w487, y="No_Test") -> (x != y?=w383:bool)
        n291 = call-poly <vilib>:"NT Read Value.vi"("Name"="Robot_Mode") -> ("String"=w406:string)  [unwired: 9 in, 1 out]
        n292 = local read "Intake_On"() -> (→"Ret_Ball_Left" →"Ret_Ball_Right":bool)
        n293 = local read "Hide_Popups"() -> (w278:bool)
        n294 = call-poly <vilib>:"NT Read Value.vi"("Name"="Feeder_Auto_Target") -> ("Boolean"=→"Ret_Feeder_Right" →"Ret_Feeder_Left":bool)  [unwired: 9 in, 1 out]
        n295 = And(x=w814, y=w813) -> (x .and. y?=w397:bool)
        n296 = call "BlinkLight.vi"() -> ("Blinked"=w575:bool)  [unwired: 1 in]
        n297 = call "EdgeTrigger.vi"("Input Signal"="Mute_Audible_Warnings") -> ("Rising Edge Trigger"=w284:bool)  [unwired: 2 out]
        n298 = Equal?(x=w406, y="Teleop Enabled") -> (x = y?=w404:bool)
        n299 = local read "Arm_Climber"() -> (w625:bool)
        n300 = call-poly <vilib>:"NT Read Value.vi"("Name"="Confirmed_States") -> ("Boolean Array"=w761:bool[])  [unwired: 9 in, 1 out]
        n301 = call-poly <vilib>:"NT Read Value.vi"("Name"="Disallowed_States") -> ("Boolean Array"=w758:bool[])  [unwired: 9 in, 1 out]
        n302 = call-poly <vilib>:"NT Read Value.vi"("Name"="Tablet_Override") -> ("Boolean"=→"Tablet_Override":bool)  [unwired: 9 in, 1 out]
        n303 = Build Array(w264, w264, w264, w271, w270, w264, w264, w264, w264, w264, w264, w264, w264, w264, w264, w264, w264, w264, w264, w264, w264) -> (w247:bool[])
        n304 = Select(t=w575, s=w459, f=TRUE) -> (s? t:f=w289:bool)
        n305 = And(x="Master_Safety_Override_1", y="Master_Safety_Override_2") -> (x .and. y?=w660:bool)
        n306 = call "EdgeTrigger.vi"("Input Signal"=w404) -> ("Rising Edge Trigger"=w403:bool)  [unwired: 2 out]
        n307 = Or(x="Error_Help", y="Driver_Help") -> (x .or. y?=w241:bool)
        n308 = Not(x=w278) -> (.not. x?=w277:bool)
        n309 = call-poly <vilib>:"NT Write Value.vi"("Boolean"=w660, "Name"="Master_Safety_Override") -> ()  [unwired: 9 in, 1 out]
        n310 = call-poly <vilib>:"NT Write Value.vi"("Boolean"="Clear_Errors", "Name"="Clear_Errors") -> ()  [unwired: 9 in, 1 out]
        n311 = call-poly <vilib>:"NT Write Value.vi"("Boolean"="Super_Test_Mode", "Name"="Super_Test_Mode") -> ()  [unwired: 9 in, 1 out]
        n312 = call-poly <vilib>:"NT Write Value.vi"("Boolean"="Camera_Override", "Name"="Camera_Override") -> ()  [unwired: 9 in, 1 out]
        n313 = call-poly <vilib>:"NT Write Value.vi"("Boolean"="Turret_Override", "Name"="Turret_Override") -> ()  [unwired: 9 in, 1 out]
        n314 = call-poly <vilib>:"NT Write Value.vi"("Boolean"="Auto_Target_Override", "Name"="Auto_Target_Override") -> ()  [unwired: 9 in, 1 out]
        n315 = call-poly <vilib>:"NT Write Value.vi"("Boolean"="Emergency_Cowl_Retract", "Name"="Emergency_Cowl_Retract") -> ()  [unwired: 9 in, 1 out]
        n316 = Initialize Array(FALSE, 20 ("dimension size")) -> (w243:bool[])
        n317 = Select(t=w289, s=w283, f=FALSE) -> (s? t:f=→"Ret_Power_Port_Left" →"Ret_Power_Port_Right":bool)
        n318 = And(x="State_Climb", y="Arm_Climber") -> (x .and. y?=w545:bool)
        n319 = And(x=w277, y=w241) -> (x .and. y?=w242:bool)
        n320 = feedback #3(TRUE ("t")) -> (w398:bool)
        n321 = Not(x=w398) -> (.not. x?=w399:bool)
        n322 = Select(t=w399, s=w284, f=w398) -> (s? t:f=w410:bool)
        n323 = Index Array(array=w758, index #1=0 ("index")) -> (element #1=w756:bool, element #2=w753:bool, element #3=w539:bool, element #4=w544:bool)  [unwired: 3 in]
        n324 = Index Array(array=w761, index #1=0 ("index")) -> (element #1=w757:bool, element #2=w754:bool, element #3=w540:bool, element #4=w543:bool)  [unwired: 3 in]
        n325 = Not(x=w625) -> (.not. x?=w621:bool)
        n326 = Select(t=TRUE, s=w403, f=w410) -> (s? t:f=w402:bool)
        "Audible_Warnings_Enabled" <- w402
        n327 = feedback-in #3(w402) -> ()
        n328 = Bundle(w397, "Super_Test_Mode"=w396, "Slow_Loop"=w395, "Drive_Train_Overheat"=w394, "Pressure_Leak"=w393, "Drive_Train_Azimuth"=w392, "Arm_Calibrate"=w391, "Auto_Error"=w390, "Auto_Test_Mode"=w389, "Shooter_Overheat"=w388, "Shooter_Motor_Failure"=w387, "Intake_Overheat"=w386, "Turret_Azimuth_Failure"=w385, "Arm_Calibrate_Turret"=w384, w383, "IMU_Failure"=w382, "Electrical_Fault"=w381, "Arm_Calibrate_Joysticks"=w380, "CAN_Bus_Fault"=w379, "Drive_Train_Shifter"=w311, "Drive_Train_Azimuth_Sensor"=w279, "Battery_Critical"=w276) -> (w378:T20)  [unwired: 1 in]
        n329 = Build Array("State_Normal", "State_Rotation_Control", "State_Position_Control", w545) -> (w764:bool[])
        n330 = call "RenderJoystickDiagram.vi"() -> ("Image Out"=w232:T3)  [unwired: 11 in]
        n331 = call "RenderRobotSystemsDiagram.vi"("Enable"=w242, "Cautions"=w247, "Nominals"=w243, "Alarms"=w246) -> ("Robot Systems Diagram"=w231:T3)  [unwired: 1 in]
        n332 = property on="Help Graphic" class="ImageControl"("Visible"=w242) -> ()  [unwired: 2 in, 2 out]
        n333 = Cluster To Array(cluster=w378) -> (array=w370:bool[])
        n334 = Sort 1D Array(array=w370) -> (sorted array=w373:bool[])
        n335 = Search 1D Array(1D array=w373, element=TRUE, start index (0)=0) -> (index of element=w367:i32)
        n336 = Array Size(array=w373) -> (size(s)=w371:i32)
        n337 = Equal?(x=w367, y=-1) -> (x = y?=w374:bool)
        n338 = Select(t=w371, s=w374, f=w367) -> (s? t:f=w372:i32)
        n339 = Subtract(x=w371, y=w372) -> (x-y=w368:i32)
        n340 = Number To Decimal String(number=w368) -> (decimal integer string=w369:string)  [unwired: 1 in]
        n341 = Or(x=w544, y=w621) -> (x .or. y?=w626:bool)
        n342 = call "BlinkLight.vi"() -> ("Blinked"=w816:bool)  [unwired: 1 in]
        n343 = Concatenate Strings("MASTER CAUTION ALARM (" ("string"), w369, ")" ("string")) -> (w364:string)
        n344 = Or Array Elements(Boolean array=w370) -> (logical OR=w361:bool)
        n345 = call "ButtonColorChooser.vi"("Un-selected Color"=w541, "Disallowed"=w756, "Confirmed"=w757) -> ("Final Color"=w755:cluster{u32, u32}[])  [unwired: 8 in]
        n346 = call "ButtonColorChooser.vi"("Un-selected Color"=w541, "Disallowed"=w753, "Confirmed"=w754) -> ("Final Color"=w751:cluster{u32, u32}[])  [unwired: 8 in]
        n347 = call "ButtonColorChooser.vi"("Un-selected Color"=w541, "Disallowed"=w626, "Confirmed"=w543) -> ("Final Color"=w752:cluster{u32, u32}[])  [unwired: 8 in]
        n348 = call "ButtonColorChooser.vi"("Un-selected Color"=w541, "Disallowed"=w539, "Confirmed"=w540) -> ("Final Color"=w542:cluster{u32, u32}[])  [unwired: 8 in]
        n349 = property on="Actuator Testing" class="Ring (strict)"() -> ("RingText.Text"=w494:string)  [unwired: 2 in, 2 out]
        n350 = call-poly <vilib>:"NT Write Value.vi"("Boolean Array"=w764, "Name"="DS_States") -> ()  [unwired: 9 in, 1 out]
        n351 = Select(t=w232, s="Driver_Help", f=w231) -> (s? t:f=→"Help Graphic":T3)
        n352 = Build Array("No_Test") -> (w491:string[])
        n353 = Select(t=w816, s=w361, f=FALSE) -> (s? t:f=w360:bool)
        "Master_Caution_1" <- w360
        "Master_Caution_0" <- w360
        "Master_Caution_2" <- w360
        n354 = Select(t=w364, s=w360, f="") -> (s? t:f=w363:string)
        n355 = property on="State_Normal" class="Bool"("Colors [4]"=w755) -> ()  [unwired: 2 in, 2 out]
        n356 = property on="State_Climb" class="Bool"("Colors [4]"=w752) -> ()  [unwired: 2 in, 2 out]
        n357 = property on="State_Rotation_Control" class="Bool"("Colors [4]"=w751) -> ()  [unwired: 2 in, 2 out]
        n358 = Select(t=cluster{u32, u32}[] [{6618880, 16448250}, {16448250, 16448250}] ("Colors [4]"), s=w402, f=cluster{u32, u32}[] [{16755474, 16448250}, {16448250, 16448250}] ("Colors [4]")) -> (s? t:f=w411:cluster{u32, u32}[])
        n359 = property on="State_Position_Control" class="Bool"("Colors [4]"=w542) -> ()  [unwired: 2 in, 2 out]
        n360 = property on="Master_Caution_0" class="Bool (strict)"("BoolText.Text"=w363) -> ()  [unwired: 2 in, 2 out]
        n361 = property on="Master_Caution_1" class="Bool (strict)"("BoolText.Text"=w363) -> ()  [unwired: 2 in, 2 out]
        n362 = property on="Master_Caution_2" class="Bool (strict)"("BoolText.Text"=w363) -> ()  [unwired: 2 in, 2 out]
        n363 = property on="Mute_Audible_Warnings" class="Bool"("Colors [4]"=w411) -> ()  [unwired: 2 in, 2 out]
        n364 = call-poly <vilib>:"NT Read Value.vi"("Default Value"=w491, "Name"="Legal_Actuator_Names") -> ("String Array"=w493:string[])  [unwired: 8 in, 1 out]
        n365 = call-poly <vilib>:"NT Write Value.vi"("String"=w494, "Name"="Test_Actuator_Name") -> ()  [unwired: 9 in, 1 out]
        n366 = call-poly <vilib>:"NT Write Value.vi"("Numeric"="Test_Actuator_Value", "Name"="Test_Actuator_Value") -> ()  [unwired: 9 in, 1 out]
        n367 = property on="Actuator Testing" class="Ring (strict)"("Strings []"=w493) -> ()  [unwired: 2 in, 2 out]
        n368 = call-poly <vilib>:"NT Write Value.vi"("Boolean"="Pre_Spin", "Name"="Pre_Spin") -> ()  [unwired: 9 in, 1 out]
        n369 = call-poly <vilib>:"NT Write Value.vi"("Boolean"="Clear_Jams", "Name"="Clear_Jams") -> ()  [unwired: 9 in, 1 out]
        n370 = call-poly <vilib>:"NT Write Value.vi"("Boolean"=w361, "Name"="Master_Caution") -> ()  [unwired: 9 in, 1 out]
        n371 = call-poly <vilib>:"NT Write Value.vi"("Numeric"="Test_Actuator_Period", "Name"="Test_Actuator_Period") -> ()  [unwired: 9 in, 1 out]
        n372 = Select(t=T13."Disabled and Grayed Out" ("Disabled"), s="Error_Help", f=T13."Enabled" ("Disabled")) -> (s? t:f=w235:T13)
        n373 = Select(t=T13."Disabled and Grayed Out" ("Disabled"), s="Driver_Help", f=T13."Enabled" ("Disabled")) -> (s? t:f=w238:T13)
        n374 = property on="Driver_Help" class="Bool (strict)"("DisabledEnum"=w235) -> ()  [unwired: 2 in, 2 out]
        n375 = property on="Error_Help" class="Bool (strict)"("DisabledEnum"=w238) -> ()  [unwired: 2 in, 2 out]
        n376 = call-poly <vilib>:"NT Read Value.vi"("Default Value"=bool[] [FALSE, FALSE, FALSE, FALSE], "Name"="Shifter_Faults") -> ("Boolean Array"=w253:bool[])  [unwired: 8 in, 1 out]
        "Shifter_Faults_Array" <- w253
        n377 = call-poly <vilib>:"NT Read Value.vi"("Default Value"=w222, "Name"="Module_Faults") -> ("Boolean Array"=w224:bool[])  [unwired: 8 in, 1 out]
        n378 = call-poly <vilib>:"NT Read Value.vi"("Name"="Drive_Overheat") -> ("Boolean Array"=w697:bool[])  [unwired: 9 in, 1 out]
        "Drive_Overheat_Array" <- w697
        n379 = call-poly <vilib>:"NT Read Value.vi"("Default Value"=w222, "Name"="Swerve_Azimuth_Sensor_Fault") -> ("Boolean Array"=w221:bool[])  [unwired: 8 in, 1 out]
        n380 = call-poly <vilib>:"NT Read Value.vi"("Name"="Field_Oriented") -> ("Boolean"=→"Field_Oriented":bool)  [unwired: 9 in, 1 out]
        n381 = call-poly <vilib>:"NT Read Value.vi"("Name"="IMU_Failure") -> ("Boolean"=→"IMU_Failure":bool)  [unwired: 9 in, 1 out]
        n382 = call-poly <vilib>:"NT Read Value.vi"("Name"="Wheel_0S_Temp") -> ("Numeric"=→"Wheel_0S_Temp":dbl)  [unwired: 9 in, 1 out]
        n383 = call-poly <vilib>:"NT Read Value.vi"("Name"="Wheel_0_Azimuth") -> ("Numeric"=→"Wheel_0_Azimuth":dbl)  [unwired: 9 in, 1 out]
        n384 = call-poly <vilib>:"NT Read Value.vi"("Name"="Wheel_0S_Velocity") -> ("Numeric"=→"Wheel_0S_Velocity":dbl)  [unwired: 9 in, 1 out]
        n385 = call-poly <vilib>:"NT Read Value.vi"("Name"="Wheel_1S_Temp") -> ("Numeric"=→"Wheel_1S_Temp":dbl)  [unwired: 9 in, 1 out]
        n386 = call-poly <vilib>:"NT Read Value.vi"("Name"="Wheel_1_Azimuth") -> ("Numeric"=→"Wheel_1_Azimuth":dbl)  [unwired: 9 in, 1 out]
        n387 = call-poly <vilib>:"NT Read Value.vi"("Name"="Wheel_1S_Velocity") -> ("Numeric"=→"Wheel_1S_Velocity":dbl)  [unwired: 9 in, 1 out]
        n388 = call-poly <vilib>:"NT Read Value.vi"("Name"="Wheel_2S_Temp") -> ("Numeric"=→"Wheel_2S_Temp":dbl)  [unwired: 9 in, 1 out]
        n389 = call-poly <vilib>:"NT Read Value.vi"("Name"="Wheel_2_Azimuth") -> ("Numeric"=→"Wheel_2_Azimuth":dbl)  [unwired: 9 in, 1 out]
        n390 = call-poly <vilib>:"NT Read Value.vi"("Name"="Wheel_2S_Velocity") -> ("Numeric"=→"Wheel_2S_Velocity":dbl)  [unwired: 9 in, 1 out]
        n391 = call-poly <vilib>:"NT Read Value.vi"("Name"="Wheel_3S_Temp") -> ("Numeric"=→"Wheel_3S_Temp":dbl)  [unwired: 9 in, 1 out]
        n392 = call-poly <vilib>:"NT Read Value.vi"("Name"="Wheel_3_Azimuth") -> ("Numeric"=→"Wheel_3_Azimuth":dbl)  [unwired: 9 in, 1 out]
        n393 = call-poly <vilib>:"NT Read Value.vi"("Name"="Wheel_3S_Velocity") -> ("Numeric"=→"Wheel_3S_Velocity":dbl)  [unwired: 9 in, 1 out]
        n394 = call-poly <vilib>:"NT Read Value.vi"("Default Value"=string[] ["U", "U", "U", "U"], "Name"="Shifter_States") -> ("String Array"=w330:string[])  [unwired: 8 in, 1 out]
        n395 = Index Array(array=w330) -> (element #1=w220:string, element #2=w219:string, element #3=w218:string, element #4=w217:string)  [unwired: 4 in]
        "Wheel_0_Shifter_State" <- w220
        "Wheel_1_Shifter_State" <- w219
        "Wheel_2_Shifter_State" <- w218
        "Wheel_3_Shifter_State" <- w217
        n396 = Or(x=w224, y=w221) -> (x .or. y?=w225:bool[])
        "Azimuth_Error_Array" <- w225
        n397 = Index Array(array=w253) -> (element #1=w313:bool, element #2=w314:bool, element #3=w315:bool, element #4=w316:bool)  [unwired: 4 in]
        n398 = Index Array(array=w697) -> (element #1=w663:bool, element #2=w678:bool, element #3=w679:bool, element #4=w680:bool)  [unwired: 4 in]
        n399 = Index Array(array=w225) -> (element #1=w229:bool, element #2=w228:bool, element #3=w227:bool, element #4=w226:bool)  [unwired: 4 in]
        n400 = Or Array Elements(Boolean array=w221) -> (logical OR=→"Drive_Train_Azimuth_Sensor":bool)
        n401 = Or Array Elements(Boolean array=w224) -> (logical OR=→"Drive_Train_Azimuth":bool)
        n402 = Compound Arithmetic op=OR(w313, w314, w315, w316) -> (→"Drive_Train_Shifter":bool)
        n403 = Compound Arithmetic op=OR(w663, w678, w679, w680) -> (→"Drive_Train_Overheat":bool)
        n404 = Equal?(x=w216, y=w220) -> (x = y?=→"High_Gear_0":bool)
        n405 = Equal?(x=w216, y=w219) -> (x = y?=→"High_Gear_1":bool)
        n406 = Equal?(x=w216, y=w218) -> (x = y?=→"High_Gear_2":bool)
        n407 = Equal?(x=w216, y=w217) -> (x = y?=→"High_Gear_3":bool)
        n408 = Select(t=u32 16711680 ("Numeric Text.Text Colors:Text Color"), s=w313, f=u32 4934475 ("Numeric Text.Text Colors:Text Color")) -> (s? t:f=w326:u32)
        n409 = Select(t=u32 16711680 ("Numeric Text.Text Colors:Text Color"), s=w314, f=u32 4934475 ("Numeric Text.Text Colors:Text Color")) -> (s? t:f=w323:u32)
        n410 = Select(t=u32 16711680 ("Numeric Text.Text Colors:Text Color"), s=w315, f=u32 4934475 ("Numeric Text.Text Colors:Text Color")) -> (s? t:f=w320:u32)
        n411 = Select(t=u32 16711680 ("Numeric Text.Text Colors:Text Color"), s=w316, f=u32 4934475 ("Numeric Text.Text Colors:Text Color")) -> (s? t:f=w317:u32)
        n412 = Select(t=u32 16711680 ("Numeric Text.Text Colors:Text Color"), s=w229, f=u32 4934475 ("Numeric Text.Text Colors:Text Color")) -> (s? t:f=w673:u32)
        n413 = Select(t=u32 16711680 ("Numeric Text.Text Colors:Text Color"), s=w228, f=u32 4934475 ("Numeric Text.Text Colors:Text Color")) -> (s? t:f=w670:u32)
        n414 = Select(t=u32 16711680 ("Numeric Text.Text Colors:Text Color"), s=w663, f=u32 4934475 ("Numeric Text.Text Colors:Text Color")) -> (s? t:f=w694:u32)
        n415 = Select(t=u32 16711680 ("Numeric Text.Text Colors:Text Color"), s=w227, f=u32 4934475 ("Numeric Text.Text Colors:Text Color")) -> (s? t:f=w667:u32)
        n416 = Select(t=u32 16711680 ("Numeric Text.Text Colors:Text Color"), s=w226, f=u32 4934475 ("Numeric Text.Text Colors:Text Color")) -> (s? t:f=w664:u32)
        n417 = Select(t=u32 16711680 ("Numeric Text.Text Colors:Text Color"), s=w678, f=u32 4934475 ("Numeric Text.Text Colors:Text Color")) -> (s? t:f=w691:u32)
        n418 = Select(t=u32 16711680 ("Numeric Text.Text Colors:Text Color"), s=w679, f=u32 4934475 ("Numeric Text.Text Colors:Text Color")) -> (s? t:f=w688:u32)
        n419 = Select(t=u32 16711680 ("Numeric Text.Text Colors:Text Color"), s=w680, f=u32 4934475 ("Numeric Text.Text Colors:Text Color")) -> (s? t:f=w685:u32)
        n420 = property on="Wheel_0_Shifter_State" class="Str"("Text.BG Color"=w326) -> ()  [unwired: 2 in, 2 out]
        n421 = property on="Wheel_1_Shifter_State" class="Str"("Text.BG Color"=w323) -> ()  [unwired: 2 in, 2 out]
        n422 = property on="Wheel_2_Shifter_State" class="Str"("Text.BG Color"=w320) -> ()  [unwired: 2 in, 2 out]
        n423 = property on="Wheel_3_Shifter_State" class="Str"("Text.BG Color"=w317) -> ()  [unwired: 2 in, 2 out]
        n424 = property on="Wheel_0S_Temp" class="DigNum (strict)"("NumText.BG Color"=w694) -> ()  [unwired: 2 in, 2 out]
        n425 = property on="Wheel_1S_Temp" class="DigNum (strict)"("NumText.BG Color"=w691) -> ()  [unwired: 2 in, 2 out]
        n426 = property on="Wheel_2S_Temp" class="DigNum (strict)"("NumText.BG Color"=w688) -> ()  [unwired: 2 in, 2 out]
        n427 = property on="Wheel_3S_Temp" class="DigNum (strict)"("NumText.BG Color"=w685) -> ()  [unwired: 2 in, 2 out]
        n428 = property on="Wheel_0_Azimuth" class="DigNum (strict)"("NumText.BG Color"=w673) -> ()  [unwired: 2 in, 2 out]
        n429 = property on="Wheel_1_Azimuth" class="DigNum (strict)"("NumText.BG Color"=w670) -> ()  [unwired: 2 in, 2 out]
        n430 = property on="Wheel_2_Azimuth" class="DigNum (strict)"("NumText.BG Color"=w667) -> ()  [unwired: 2 in, 2 out]
        n431 = property on="Wheel_3_Azimuth" class="DigNum (strict)"("NumText.BG Color"=w664) -> ()  [unwired: 2 in, 2 out]
        n432 = call-poly <vilib>:"NT Read Value.vi"("Name"="Shoot_Overheat") -> ("Boolean Array"=w648:bool[])  [unwired: 9 in, 1 out]
        n433 = call-poly <vilib>:"NT Read Value.vi"("Name"="Cowl_State") -> ("String"=w551:string)  [unwired: 9 in, 1 out]
        n434 = call-poly <vilib>:"NT Read Value.vi"("Name"="Out_Of_Range") -> ("Boolean"=→"Out_Of_Range":bool)  [unwired: 9 in, 1 out]
        n435 = call-poly <vilib>:"NT Read Value.vi"("Name"="Ready_To_Shoot") -> ("Boolean"=→"Ready_To_Shoot":bool)  [unwired: 9 in, 1 out]
        n436 = call-poly <vilib>:"NT Read Value.vi"("Name"="Shooter_Motor_Failure") -> ("Boolean Array"=w585:bool[])  [unwired: 9 in, 1 out]
        n437 = call-poly <vilib>:"NT Read Value.vi"("Default Value"=0.0, "Name"="Balls_Shot") -> ("Numeric"=w469:dbl)  [unwired: 8 in, 1 out]
        n438 = call-poly <vilib>:"NT Read Value.vi"("Name"="Shooter_Power") -> ("Numeric"=→"Shooter_Power":dbl)  [unwired: 9 in, 1 out]
        n439 = call-poly <vilib>:"NT Read Value.vi"("Name"="Retrieved_Kicker_Power") -> ("Numeric"=→"Kicker_Power":dbl)  [unwired: 9 in, 1 out]
        n440 = call-poly <vilib>:"NT Read Value.vi"("Name"="Shooter_0_RPM_Actual") -> ("Numeric"=w633:dbl)  [unwired: 9 in, 1 out]
        "Shooter_0_RPM_Actual_Detail" <- w633
        n441 = call-poly <vilib>:"NT Read Value.vi"("Name"="Shooter_1_RPM_Actual") -> ("Numeric"=w632:dbl)  [unwired: 9 in, 1 out]
        "Shooter_1_RPM_Actual_Detail" <- w632
        n442 = call-poly <vilib>:"NT Read Value.vi"("Name"="Kicker_RPM_Actual") -> ("Numeric"=→"Kicker_RPM_Actual_Detail":dbl)  [unwired: 9 in, 1 out]
        n443 = call-poly <vilib>:"NT Read Value.vi"("Name"="Shooter_RPM_Goal") -> ("Numeric"=→"Shooter_RPM_Goal" →"Shooter_RPM_Goal_Detail":dbl)  [unwired: 9 in, 1 out]
        n444 = call-poly <vilib>:"NT Read Value.vi"("Name"="Kicker_RPM_Goal") -> ("Numeric"=→"Kicker_RPM_Goal_Detail":dbl)  [unwired: 9 in, 1 out]
        n445 = call-poly <vilib>:"NT Read Value.vi"("Name"="Shooter_0_Temp") -> ("Numeric"=→"Shooter_0_Temp":dbl)  [unwired: 9 in, 1 out]
        n446 = call-poly <vilib>:"NT Read Value.vi"("Name"="Shooter_1_Temp") -> ("Numeric"=→"Shooter_1_Temp":dbl)  [unwired: 9 in, 1 out]
        n447 = call-poly <vilib>:"NT Read Value.vi"("Name"="Kicker_Temp") -> ("Numeric"=→"Kicker_Temp":dbl)  [unwired: 9 in, 1 out]
        n448 = To Long Integer(number=w469) -> (32bit integer=→"Balls_Shot":i32)
        n449 = call-poly <vilib>:"NT Read Value.vi"("Name"="Confirmed_ShooterModes") -> ("Boolean Array"=w614:bool[])  [unwired: 9 in, 1 out]
        n450 = call-poly <vilib>:"NT Read Value.vi"("Name"="Disallowed_ShooterModes") -> ("Boolean Array"=w611:bool[])  [unwired: 9 in, 1 out]
        n451 = call-poly <vilib>:"NT Read Value.vi"("Name"="Beam_Break_Raw") -> ("Numeric"=w356:dbl)  [unwired: 9 in, 1 out]
        n452 = call-poly <vilib>:"NT Read Value.vi"("Name"="LIDAR_Distance_To_Target") -> ("Numeric"=→"LIDAR_Distance_To_Target":dbl)  [unwired: 9 in, 1 out]
        n453 = Index Array(array=w648) -> (element #1=w640:bool, element #2=w641:bool, element #3=w531:bool)  [unwired: 3 in]
        n454 = Equal?(x="A", y=w551) -> (x = y?=→"Cowl_A":bool)
        n455 = Equal?(x="B", y=w551) -> (x = y?=→"Cowl_B":bool)
        n456 = Equal?(x="C", y=w551) -> (x = y?=→"Cowl_C":bool)
        n457 = Index Array(array=w585) -> (element #1=w577:bool, element #2=w578:bool)  [unwired: 2 in]
        n458 = Compound Arithmetic op=ADD(w633, w632) -> (w631:dbl)
        n459 = To Long Integer(number=w356) -> (32bit integer=→"Beam_Break_Raw":i32)
        n460 = Build Array("Mode_TargetingComputer", "Mode_Wall", "Mode_InitiationLine", "Mode_CloseTrench", "Mode_FarTrench") -> (w623:bool[])
        n461 = Divide(x=w631, y=2.0) -> (x/y=→"Shooter_RPM_Actual":dbl)
        n462 = Index Array(array=w611, index #1=0 ("index")) -> (element #1=w609:bool, element #2=w606:bool, element #3=w602:bool, element #4=w597:bool, element #5=w596:bool)  [unwired: 4 in]
        n463 = Index Array(array=w614, index #1=0 ("index")) -> (element #1=w610:bool, element #2=w607:bool, element #3=w605:bool, element #4=w599:bool, element #5=w598:bool)  [unwired: 4 in]
        n464 = Compound Arithmetic op=OR(w640, w641, w531) -> (→"Shooter_Overheat":bool)
        n465 = Select(t=u32 16711680 ("Numeric Text.Text Colors:Text Color"), s=w640, f=u32 4934475 ("Numeric Text.Text Colors:Text Color")) -> (s? t:f=w645:u32)
        n466 = Compound Arithmetic op=OR(w577, w578) -> (→"Shooter_Motor_Failure":bool)
        n467 = Select(t=u32 16711680 ("Numeric Text.Text Colors:Text Color"), s=w641, f=u32 4934475 ("Numeric Text.Text Colors:Text Color")) -> (s? t:f=w642:u32)
        n468 = Select(t=u32 16711680 ("Numeric Text.Text Colors:Text Color"), s=w531, f=u32 4934475 ("Numeric Text.Text Colors:Text Color")) -> (s? t:f=w532:u32)
        n469 = Select(t=u32 16711680 ("Numeric Text.Text Colors:Text Color"), s=w577, f=u32 4934475 ("Numeric Text.Text Colors:Text Color")) -> (s? t:f=w582:u32)
        n470 = Select(t=u32 16711680 ("Numeric Text.Text Colors:Text Color"), s=w578, f=u32 4934475 ("Numeric Text.Text Colors:Text Color")) -> (s? t:f=w579:u32)
        n471 = call-poly <vilib>:"NT Write Value.vi"("Boolean Array"=w623, "Name"="Shooter_Modes") -> ()  [unwired: 9 in, 1 out]
        n472 = property on="Shooter_0_Temp" class="DigNum (strict)"("NumText.BG Color"=w645) -> ()  [unwired: 2 in, 2 out]
        n473 = property on="Shooter_1_Temp" class="DigNum (strict)"("NumText.BG Color"=w642) -> ()  [unwired: 2 in, 2 out]
        n474 = property on="Kicker_Temp" class="DigNum (strict)"("NumText.BG Color"=w532) -> ()  [unwired: 2 in, 2 out]
        n475 = property on="Shooter_0_RPM_Actual_Detail" class="DigNum (strict)"("NumText.BG Color"=w582) -> ()  [unwired: 2 in, 2 out]
        n476 = property on="Shooter_1_RPM_Actual_Detail" class="DigNum (strict)"("NumText.BG Color"=w579) -> ()  [unwired: 2 in, 2 out]
        n477 = call "ButtonColorChooser.vi"("Un-selected Color"=w595, "Disallowed"=w609, "Confirmed"=w610) -> ("Final Color"=w608:cluster{u32, u32}[])  [unwired: 8 in]
        n478 = call "ButtonColorChooser.vi"("Un-selected Color"=w595, "Disallowed"=w606, "Confirmed"=w607) -> ("Final Color"=w603:cluster{u32, u32}[])  [unwired: 8 in]
        n479 = call "ButtonColorChooser.vi"("Un-selected Color"=w595, "Disallowed"=w602, "Confirmed"=w605) -> ("Final Color"=w604:cluster{u32, u32}[])  [unwired: 8 in]
        n480 = call "ButtonColorChooser.vi"("Un-selected Color"=w595, "Disallowed"=w597, "Confirmed"=w599) -> ("Final Color"=w601:cluster{u32, u32}[])  [unwired: 8 in]
        n481 = call "ButtonColorChooser.vi"("Un-selected Color"=w595, "Disallowed"=w596, "Confirmed"=w598) -> ("Final Color"=w600:cluster{u32, u32}[])  [unwired: 8 in]
        n482 = property on="Mode_TargetingComputer" class="Bool"("Colors [4]"=w608) -> ()  [unwired: 2 in, 2 out]
        n483 = property on="Mode_InitiationLine" class="Bool"("Colors [4]"=w604) -> ()  [unwired: 2 in, 2 out]
        n484 = property on="Mode_CloseTrench" class="Bool"("Colors [4]"=w601) -> ()  [unwired: 2 in, 2 out]
        n485 = property on="Mode_FarTrench" class="Bool"("Colors [4]"=w600) -> ()  [unwired: 2 in, 2 out]
        n486 = property on="Mode_Wall" class="Bool"("Colors [4]"=w603) -> ()  [unwired: 2 in, 2 out]
        n487 = call-poly <vilib>:"NT Read Value.vi"("Name"="Intake_On") -> ("Boolean"=→"Intake_On":bool)  [unwired: 9 in, 1 out]
        n488 = call-poly <vilib>:"NT Read Value.vi"("Name"="Flapper_Flapping") -> ("Boolean"=→"Flapper_Flapping":bool)  [unwired: 9 in, 1 out]
        n489 = call-poly <vilib>:"NT Read Value.vi"("Name"="Intake_Temp") -> ("Numeric"=→"Intake_Temp":dbl)  [unwired: 9 in, 1 out]
        n490 = call-poly <vilib>:"NT Read Value.vi"("Name"="Climber_Climbing") -> ("Boolean"=→"Climber_Climbing":bool)  [unwired: 9 in, 1 out]
        n491 = call-poly <vilib>:"NT Read Value.vi"("Name"="Intake_Overheat") -> ("Boolean"=w513:bool)  [unwired: 9 in, 1 out]
        "Intake_Overheat" <- w513
        n492 = call-poly <vilib>:"NT Read Value.vi"("Name"="Turret_Azimuth") -> ("Numeric"=→"Turret_Azimuth":dbl)  [unwired: 9 in, 1 out]
        n493 = call-poly <vilib>:"NT Read Value.vi"("Name"="Turret_Azimuth_Failure") -> ("Boolean"=w498:bool)  [unwired: 9 in, 1 out]
        "Turret_Azimuth_Failure" <- w498
        n494 = call-poly <vilib>:"NT Read Value.vi"("Name"="Turret_Limit_Switch_A") -> ("Boolean"=→"Turret_Limit_Switch_A":bool)  [unwired: 9 in, 1 out]
        n495 = call-poly <vilib>:"NT Read Value.vi"("Name"="Turret_Limit_Switch_B") -> ("Boolean"=→"Turret_Limit_Switch_B":bool)  [unwired: 9 in, 1 out]
        n496 = Select(t=u32 16711680 ("Numeric Text.Text Colors:Text Color"), s=w513, f=u32 4934475 ("Numeric Text.Text Colors:Text Color")) -> (s? t:f=w514:u32)
        n497 = Select(t=u32 16711680 ("Numeric Text.Text Colors:Text Color"), s=w498, f=u32 4934475 ("Numeric Text.Text Colors:Text Color")) -> (s? t:f=w499:u32)
        n498 = property on="Intake_Temp" class="DigNum (strict)"("NumText.BG Color"=w514) -> ()  [unwired: 2 in, 2 out]
        n499 = property on="Turret_Azimuth" class="DigNum (strict)"("NumText.BG Color"=w499) -> ()  [unwired: 2 in, 2 out]
        n500 = And(x="Calibrate_Turret", y="Arm_Calibrate_Turret") -> (x .and. y?=w508:bool)
        n501 = And(x="Calibrate_Wheels", y="Arm_Calibrate") -> (x .and. y?=w656:bool)
        n502 = Not(x="Arm_Calibrate") -> (.not. x?=w458:bool)
        n503 = Not(x="Arm_Calibrate_Turret") -> (.not. x?=w505:bool)
        n504 = call-poly <vilib>:"NT Write Value.vi"("Boolean"="Zero_Wheels", "Name"="Zero_Wheels") -> ()  [unwired: 9 in, 1 out]
        n505 = call-poly <vilib>:"NT Write Value.vi"("Boolean"=w656, "Name"="Calibrate_Wheels") -> ()  [unwired: 9 in, 1 out]
        n506 = call-poly <vilib>:"NT Write Value.vi"("Boolean"="Zero_Turret", "Name"="Zero_Turret") -> ()  [unwired: 9 in, 1 out]
        n507 = call-poly <vilib>:"NT Write Value.vi"("Boolean"=w508, "Name"="Calibrate_Turret") -> ()  [unwired: 9 in, 1 out]
        n508 = call-poly <vilib>:"NT Write Value.vi"("Numeric"="Wall_Speed", "Name"="Wall_Speed") -> ()  [unwired: 9 in, 1 out]
        n509 = call-poly <vilib>:"NT Write Value.vi"("Numeric"="Initiation_Line", "Name"="Initiation_Line_Speed") -> ()  [unwired: 9 in, 1 out]
        n510 = call-poly <vilib>:"NT Write Value.vi"("Numeric"="Close_Trench_Speed", "Name"="Close_Trench_Speed") -> ()  [unwired: 9 in, 1 out]
        n511 = call-poly <vilib>:"NT Write Value.vi"("Numeric"="Far_Trench_Speed", "Name"="Far_Trench_Speed") -> ()  [unwired: 9 in, 1 out]
        n512 = call-poly <vilib>:"NT Write Value.vi"("Numeric"="All_Kicker_Speed", "Name"="All_Kicker_Speed") -> ()  [unwired: 9 in, 1 out]
        n513 = Select(t=cluster{u32, u32}[] [{11776947, 16448250}, {16448250, 16448250}] ("Colors [4]"), s=w458, f=cluster{u32, u32}[] [{6618880, 16448250}, {16448250, 16448250}] ("Colors [4]")) -> (s? t:f=w559:cluster{u32, u32}[])
        n514 = Select(t=cluster{u32, u32}[] [{11776947, 16448250}, {16448250, 16448250}] ("Colors [4]"), s=w505, f=cluster{u32, u32}[] [{6618880, 16448250}, {16448250, 16448250}] ("Colors [4]")) -> (s? t:f=w504:cluster{u32, u32}[])
        n515 = property on="Calibrate_Wheels" class="Bool"("Colors [4]"=w559) -> ()  [unwired: 2 in, 2 out]
        n516 = property on="Calibrate_Turret" class="Bool"("Colors [4]"=w504) -> ()  [unwired: 2 in, 2 out]
      }
    }
  }
  n517 = vi-ref "Playback Controls.vi"() -> (w31:refnum<vi>)
  n518 = control-ref of="Command Params"() -> (w12:refnum<vi>)
  n519 = while {
    tunnel: [w884] -> _
    tunnel: w35 -> [w883]
    tunnel: w31 -> [w882]
    tunnel: w30 -> [w881]
    tunnel: w29 -> [_]
    tunnel: w25 -> [w880]
    tunnel: w13 -> [w879]
    tunnel: w12 -> [w878]
    shift-right: [w877] -> _
    shift-left: _ -> [w876]
    tunnel: w10 -> [w875]
    i -> [w884]
    stop <- FALSE stop-if-true
    n520 = event shown="[0] Timeout" {
      selector: w881 -> [_ _ _ _ _ _ _ _ _ _ _ _ _ _ _ _ _ _ _ _ _]
      dyn-events: [_ _ _ _ _ _ _ _ _ _ _ _ _ _ _ _ w1142 _ _ _ _] -> _
      timeout: u32 60 ("milliseconds to wait") -> [_ _ _ _ _ _ _ _ _ _ _ _ _ _ _ _ _ _ _ _ _]
      tunnel: w883 -> [w896 _ _ _ _ _ _ _ _ _ _ _ _ _ _ _ _ _ _ _ _]
      tunnel: "Test Tree" -> [_ _ _ _ _ _ _ _ _ _ _ w1111 w1119 w1121 w1125 w1133 _ _ _ _ _]
      tunnel: w882 -> [_ _ _ _ _ _ _ _ _ _ _ _ _ _ _ _ w1144 _ w1162 _ _]
      tunnel: w880 -> [_ _ _ _ _ _ _ _ _ _ _ _ _ _ _ _ w1140 _ _ _ _]
      tunnel: w879 -> [_ _ _ _ _ _ _ _ _ _ _ _ _ _ _ _ w1138 _ _ _ _]
      tunnel: w878 -> [w891 _ _ _ _ _ w1062 _ _ _ _ _ _ _ _ _ _ _ _ _ _]
      tunnel: [w890 w939 w1041 w1046 w1055 w1059 w1060 w1069 w1079 w1086 w1098 w1110 w1117 w1120 w1124 w1132 w1137 w1157 w1159 w1163 w1176] -> w877
      tunnel: w876 -> [w890 w939 w1041 w1046 w1055 w1059 w1060 _ _ w1086 w1098 w1110 w1117 w1120 w1124 w1132 w1137 w1157 w1159 w1163 w1176]
      tunnel: w875 -> [w888 _ _ _ _ _ _ _ _ _ _ _ _ _ _ _ _ _ _ _ _]
      event Timeout {
        n521 = event-data() -> ()  [unwired: 1 in, 1 out]
        n522 = local read "Mode"() -> (w893:T5)
        n523 = case shown="\"Commands\"" "Dashboard Tab" {
          tunnel: w896 -> [_ _ w912 _ _]
          tunnel: "TestMode/Automatic/" ("Name Pattern") -> [_ _ w911 _ _]
          tunnel: T21 [{"Operation"=enum."Clear", "Color Box"=14013909}, {"Operation"=enum."Clear", "Color Box"=14013909}, {"Operation"=enum."Clear", "Color Box"=14013909}, {"Operation"=enum."Clear", "Color Box"=14013909}, {"Operation"=enum."Update", "Color Box"=14013909}, {"Operation"=enum."Update", "Color Box"=16777215}, {"Operation"=enum."Clear", "Color Box"=14013909}, {"Operation"=enum."Clear", "Color Box"=14013909}, {"Operation"=enum."Clear", "Color Box"=14013909}] -> [_ _ w904 _ w932]
          tunnel: w893 -> [_ _ w903 _ w931]
          tunnel: u32[] [15790320, 15790320, 15790320, 15790320, 16777215, 16777215, 15790320, 15790320, 15790320] -> [_ _ _ _ w937]
          tunnel: w891 -> [_ _ _ _ w925]
          tunnel: w888 -> [_ w898 _ _ _]
          frame "TeleOp", Default {
          }
          frame "Tune" {
            n524 = call <vilib>:"WPI_DashboardUpdateNames.vi"("Controls on Tab"=w898) -> ()  [unwired: 11 in]
          }
          frame "Test" {
            w910 = -2 ("Active Item:Row Number")
            n525 = Index Array(array=w904, index=w903) -> (element=w905:T24)
            n526 = Unbundle(w905) -> ("Operation"=w906:enum16{"Update", "Clear"}, "Color Box"=w907:u32)
            n527 = call <vilib>:"NT Read String.vi"("Name"="TestMode/TestName") -> ("String"=w901:string)  [unwired: 9 in, 1 out]
            n528 = call <vilib>:"NT Read and Format Entries as Tree.vi"("Operation"=w906, "Name Pattern"=w911, "Tree Refnum"=w912) -> ()  [unwired: 7 in, 2 out]
            n529 = case shown="\"\"" w901 {
              tunnel: "TestMode/TestProgress" ("Name") -> [w914 _]
              tunnel: "TestMode/TestProgressText" ("Name") -> [w913 _]
              frame Default {
                n530 = call <vilib>:"NT Read Number.vi"("Name"=w914) -> ("Numeric"=w915:dbl)  [unwired: 9 in, 1 out]
                n531 = call <vilib>:"NT Read String.vi"("Name"=w913) -> ("String"=w916:string)  [unwired: 9 in, 1 out]
                n532 = Bundle("Numeric"=w915, "String"=w916) -> (→"Progress":cluster{"Numeric":dbl, "String":string})  [unwired: 1 in]
              }
              frame "" {
                n533 = property on="Progress" class="Clust (strict)"("Visible"=FALSE) -> ()  [unwired: 2 in, 2 out]
                n534 = local write "Test Name"(u16 0) -> ()
              }
            }
            n535 = property on="Test Tree" class="Tree (strict)"("Active Item Row Number"=w910, "ActiveColNum"=w910, "CellBG"=w907, "Active Item Row Number"=-1 ("Active Item:Row Number"), "CellBG"=u32 5789784 ("Color Box")) -> ()  [unwired: 2 in, 2 out]
          }
          frame "Variables" {
            w922 = string[] ["CameraPublisher", "Usage", "DB"]  # Items to initially close
            n536 = First Call?() -> (First Call?: T/F=w923:bool)
            n537 = control-ref of="Tree"() -> (w924:refnum<vi>)
            n538 = Select(t=w922, s=w923, f=string[] []) -> (s? t:f=w920:string[])
            n539 = call <vilib>:"NT Read and Format Entries as Tree.vi"("Tags to  Close"=w920, "Tree Refnum"=w924) -> ()  [unwired: 8 in, 2 out]
          }
          frame "Commands" {
            w933 = u32 5789784 ("Color Box")
            w934 = T25 {"Row"=-1, "Column"=-2} ("Active Cell:Active Cell")
            w936 = T25 {"Row"=-2, "Column"=-2} ("Active Cell:Active Cell")
            n540 = Index Array(array=w937, index=w931) -> (element=w935:u32)
            n541 = Index Array(array=w932, index=w931) -> (element=w930:T24)
            n542 = Unbundle(w930) -> ("Operation"=w929:enum16{"Update", "Clear"})  [unwired: 1 out]
            n543 = local read "Command Selection"() -> (w928:i32)
            n544 = property on="Command Selection" class="MCListbox (strict)"("ActiveCell"=w936, "CellBG"=w935, "ActiveCell"=w934, "CellBG"=w933) -> ()  [unwired: 2 in, 2 out]
            n545 = call <vilib>:"WPI_DashboardUpdate RPC Info.vi"("Operation"=w929) -> ("update"=w927:bool, "commands"=w926:string[][])  [unwired: 9 in]
            n546 = property on="Command Selection" class="MCListbox (strict)"("ItemNames"=w926) -> ()  [unwired: 2 in, 2 out]
            n547 = property on="Command Params" class="Tbl (strict)"("Active Cell"=w936, "Cell BG Color"=w935, "Active Cell"=w934, "Cell BG Color"=w933) -> ()  [unwired: 2 in, 2 out]
            n548 = call <vilib>:"WPI_DashboardUpdate Command Params.vi"("Update"=w927, "NewVal"=w928, "Commands"=w926, "Param Tbl"=w925) -> ()  [unwired: 7 in, 1 out]
          }
        }
        n549 = call <vilib>:"Connextion Info.vi"() -> ("Connected"=→"NT Connection":bool)  [unwired: 10 in, 1 out]
      }
      event "Test Tree": Value Change {
        # "Show appropriate\ncontrols"
        n550 = event-data() -> ("CtlRef"=w942:refnum<vi>, "NewVal"=w940:string)  [unwired: 1 in]
        n551 = call <vilib>:"WPI_UtilitiesGetTreeIOName.vi"("NewVal"=w940, "TreeControl in"=w942) -> ("I/O Name"=w943:string)  [unwired: 9 in]
        n552 = case shown="\"Analog Out\", \"Motor\", \"PWM\"" w943 {
          selector: w943 -> [_ w950 _ w972 w981 _]
          tunnel: w940 -> [_ _ w969 w971 _ w988]
          tunnel: cluster{string[]}[] [{["640x480", "320x240", "160x120"]}, {["Auto", "Fixed indoor", "Fixed outdoor 1", "Fixed outdoor 2", "Fixed fluorescent 1", "Fixed fluorescent 2", "Hold current"]}, {["Auto", "Flicker-free 50 Hz", "Flicker-free 60 Hz", "Hold current"]}, {["None", "Prioritize frame rate", "Prioritize image quality"]}, {["Monochrome", "Color"]}] -> [_ _ _ _ _ w987]
          frame Default {
            w945 = FALSE ("Visible")
            w944 = FALSE ("Visible")
            n553 = property on="Motor" class="Clust (strict)"("Visible"=w944) -> ()  [unwired: 2 in, 2 out]
            n554 = property on="Test Ring" class="Ring (strict)"("Visible"=w944) -> ()  [unwired: 2 in, 2 out]
            n555 = property on="Rev/Fwd" class="Clust (strict)"("Visible"=w945) -> ()  [unwired: 2 in, 2 out]
            n556 = property on="On/Off" class="Bool (strict)"("Visible"=w945) -> ()  [unwired: 2 in, 2 out]
            n557 = property on="Test Slider" class="Slide (strict)"("Visible"=w945) -> ()  [unwired: 2 in, 2 out]
          }
          frame "Analog Out", "Motor", "PWM" {
            w951 = FALSE ("Visible")
            n558 = case shown="\"Analog Out\"" w950 {
              tunnel: [1.0 ("Value") -1.0 ("Value") 0.0 ("Value")] -> w949
              tunnel: [255.0 ("Value") 1.0 ("Value") 5.0 ("Value")] -> w948
              tunnel: [128.0 ("Value") 0.0 ("Value") 0.0 ("Value")] -> w947
              tunnel: [64.0 ("Value") 0.5 ("Value") 1.0 ("Value")] -> w946
              frame "PWM" {
              }
              frame "Motor", Default {
              }
              frame "Analog Out" {
              }
            }
            n559 = property on="Motor" class="Clust (strict)"("Visible"=TRUE) -> ()  [unwired: 2 in, 2 out]
            n560 = property on="Value" class="Slide (strict)"("Value"=w947, "Scale.Minimum"=w949, "Scale.Maximum"=w948, "Scale.Increment"=w946) -> ()  [unwired: 2 in, 2 out]
            n561 = property on="On/Off" class="Bool (strict)"("Visible"=w951) -> ()  [unwired: 2 in, 2 out]
            n562 = property on="Test Slider" class="Slide (strict)"("Visible"=w951) -> ()  [unwired: 2 in, 2 out]
            n563 = property on="Test Ring" class="Ring (strict)"("Visible"=w951) -> ()  [unwired: 2 in, 2 out]
            n564 = property on="Rev/Fwd" class="Clust (strict)"("Visible"=w951) -> ()  [unwired: 2 in, 2 out]
          }
          frame "Servo" {
            w967 = FALSE ("Visible")
            n565 = call <vilib>:"NT Read Number.vi"("Name"=w969) -> ("Numeric"=w968:dbl)  [unwired: 9 in, 1 out]
            n566 = property on="Test Slider" class="Slide (strict)"("Visible"=TRUE, "Scale.Maximum"=170.0 ("Scale.Range:Maximum")) -> ()  [unwired: 2 in, 2 out]
            n567 = local write "Test Slider"(w968) -> ()
            n568 = property on="Motor" class="Clust (strict)"("Visible"=w967) -> ()  [unwired: 2 in, 2 out]
            n569 = property on="Rev/Fwd" class="Clust (strict)"("Visible"=w967) -> ()  [unwired: 2 in, 2 out]
            n570 = property on="On/Off" class="Bool (strict)"("Visible"=w967) -> ()  [unwired: 2 in, 2 out]
            n571 = property on="Test Ring" class="Ring (strict)"("Visible"=w967) -> ()  [unwired: 2 in, 2 out]
          }
          frame "Relay", "Solenoid" {
            w970 = FALSE ("Visible")
            n572 = property on="Motor" class="Clust (strict)"("Visible"=w970) -> ()  [unwired: 2 in, 2 out]
            n573 = property on="Test Slider" class="Slide (strict)"("Visible"=w970) -> ()  [unwired: 2 in, 2 out]
            n574 = Search and Replace String(input string=w971, search string="/Value  **", replace string="/Direction") -> (result string=w977:string)  [unwired: 5 in, 3 out]
            n575 = property on="Test Ring" class="Ring (strict)"("Visible"=w970) -> ()  [unwired: 2 in, 2 out]
            n576 = call <vilib>:"NT Read String.vi"("Name"=w977) -> ("String"=w975:string)  [unwired: 9 in, 1 out]
            n577 = Equal?(x="Both directions", y=w975) -> (x = y?=w973:bool)
            n578 = Not(x=w973) -> (.not. x?=w974:bool)
            n579 = property on="Rev/Fwd" class="Clust (strict)"("Visible"=w973) -> ()  [unwired: 2 in, 2 out]
            n580 = property on="On/Off" class="Bool (strict)"("Visible"=w974, "Caption.Text"=w972) -> ()  [unwired: 2 in, 2 out]
          }
          frame "Compressor", "Digital Out" {
            w980 = FALSE ("Visible")
            # "Get direction and finish"
            n581 = property on="Motor" class="Clust (strict)"("Visible"=w980) -> ()  [unwired: 2 in, 2 out]
            n582 = property on="Test Slider" class="Slide (strict)"("Visible"=w980) -> ()  [unwired: 2 in, 2 out]
            n583 = property on="Test Ring" class="Ring (strict)"("Visible"=w980) -> ()  [unwired: 2 in, 2 out]
            n584 = property on="On/Off" class="Bool (strict)"("Visible"=TRUE, "Caption.Text"=w981) -> ()  [unwired: 2 in, 2 out]
            n585 = property on="Rev/Fwd" class="Clust (strict)"("Visible"=FALSE) -> ()  [unwired: 2 in, 2 out]
          }
          frame "Camera" {
            n586 = call <vilib>:"Get Last Path Segment.vi"("String in"=w988) -> ("String out"=w989:string)  [unwired: 10 in]
            n587 = property on="On/Off" class="Bool (strict)"("Visible"=FALSE) -> ()  [unwired: 2 in, 2 out]
            n588 = property on="Motor" class="Clust (strict)"("Visible"=FALSE) -> ()  [unwired: 2 in, 2 out]
            n589 = property on="Rev/Fwd" class="Clust (strict)"("Visible"=FALSE) -> ()  [unwired: 2 in, 2 out]
            n590 = case shown="\"White Balance  **\"" w989 {
              tunnel: w988 -> [w995 w1004 w1013 w1022 w1031 _ w1037]
              tunnel: w987 -> [w993 w1001 w1010 w1019 w1028 _ _]
              frame "Size  **" {
                n591 = Index Array(array=w993) -> (element=w992:cluster{string[]})  [unwired: 1 in]
                n592 = call <vilib>:"NT Read String.vi"("Name"=w995) -> ("String"=w994:string)  [unwired: 9 in, 1 out]
                n593 = Unbundle(w992) -> (w990:string[])
                n594 = Match First String(2:w990, 3:w994) -> (0:w991:i32)  [unwired: 1 out]
                n595 = property on="Test Ring" class="Ring (strict)"("Value"=w991, "Strings []"=w990) -> ()  [unwired: 2 in, 2 out]
                n596 = property on="Test Ring" class="Ring (strict)"("Visible"=TRUE) -> ()  [unwired: 2 in, 2 out]
                n597 = property on="Test Slider" class="Slide (strict)"("Visible"=FALSE) -> ()  [unwired: 2 in, 2 out]
              }
              frame "White Balance  **" {
                n598 = Index Array(array=w1001, index=1) -> (element=w1002:cluster{string[]})
                n599 = call <vilib>:"NT Read String.vi"("Name"=w1004) -> ("String"=w1003:string)  [unwired: 9 in, 1 out]
                n600 = Unbundle(w1002) -> (w999:string[])
                n601 = Match First String(2:w999, 3:w1003) -> (0:w998:i32)  [unwired: 1 out]
                n602 = property on="Test Ring" class="Ring (strict)"("Value"=w998, "Strings []"=w999) -> ()  [unwired: 2 in, 2 out]
                n603 = property on="Test Ring" class="Ring (strict)"("Visible"=TRUE) -> ()  [unwired: 2 in, 2 out]
                n604 = property on="Test Slider" class="Slide (strict)"("Visible"=FALSE) -> ()  [unwired: 2 in, 2 out]
              }
              frame "Exposure  **" {
                n605 = Index Array(array=w1010, index=2) -> (element=w1011:cluster{string[]})
                n606 = call <vilib>:"NT Read String.vi"("Name"=w1013) -> ("String"=w1012:string)  [unwired: 9 in, 1 out]
                n607 = Unbundle(w1011) -> (w1007:string[])
                n608 = Match First String(2:w1007, 3:w1012) -> (0:w1008:i32)  [unwired: 1 out]
                n609 = property on="Test Ring" class="Ring (strict)"("Value"=w1008, "Strings []"=w1007) -> ()  [unwired: 2 in, 2 out]
                n610 = property on="Test Ring" class="Ring (strict)"("Visible"=TRUE) -> ()  [unwired: 2 in, 2 out]
                n611 = property on="Test Slider" class="Slide (strict)"("Visible"=FALSE) -> ()  [unwired: 2 in, 2 out]
              }
              frame "Exposure Priority  **" {
                n612 = Index Array(array=w1019, index=3) -> (element=w1020:cluster{string[]})
                n613 = call <vilib>:"NT Read String.vi"("Name"=w1022) -> ("String"=w1021:string)  [unwired: 9 in, 1 out]
                n614 = Unbundle(w1020) -> (w1016:string[])
                n615 = Match First String(2:w1016, 3:w1021) -> (0:w1017:i32)  [unwired: 1 out]
                n616 = property on="Test Ring" class="Ring (strict)"("Value"=w1017, "Strings []"=w1016) -> ()  [unwired: 2 in, 2 out]
                n617 = property on="Test Ring" class="Ring (strict)"("Visible"=TRUE) -> ()  [unwired: 2 in, 2 out]
                n618 = property on="Test Slider" class="Slide (strict)"("Visible"=FALSE) -> ()  [unwired: 2 in, 2 out]
              }
              frame "Color Enable  **" {
                n619 = Index Array(array=w1028, index=4) -> (element=w1029:cluster{string[]})
                n620 = call <vilib>:"NT Read String.vi"("Name"=w1031) -> ("String"=w1030:string)  [unwired: 9 in, 1 out]
                n621 = Unbundle(w1029) -> (w1025:string[])
                n622 = Match First String(2:w1025, 3:w1030) -> (0:w1026:i32)  [unwired: 1 out]
                n623 = property on="Test Ring" class="Ring (strict)"("Value"=w1026, "Strings []"=w1025) -> ()  [unwired: 2 in, 2 out]
                n624 = property on="Test Ring" class="Ring (strict)"("Visible"=TRUE) -> ()  [unwired: 2 in, 2 out]
                n625 = property on="Test Slider" class="Slide (strict)"("Visible"=FALSE) -> ()  [unwired: 2 in, 2 out]
              }
              frame Default {
                n626 = property on="Test Ring" class="Ring (strict)"("Visible"=FALSE) -> ()  [unwired: 2 in, 2 out]
                n627 = property on="Test Slider" class="Slide (strict)"("Visible"=FALSE) -> ()  [unwired: 2 in, 2 out]
              }
              frame "Brightness  **", "Color Level  **", "Compression  **", "FPS  **", "Sharpness  **" {
                n628 = call <vilib>:"NT Read Number.vi"("Name"=w1037) -> ("Numeric"=w1036:dbl)  [unwired: 9 in, 1 out]
                n629 = local write "Test Slider"(w1036) -> ()
                n630 = property on="Test Slider" class="Slide (strict)"("Visible"=TRUE, "Scale.Maximum"=100.0 ("Scale.Range:Maximum")) -> ()  [unwired: 2 in, 2 out]
                n631 = property on="Test Ring" class="Ring (strict)"("Visible"=FALSE) -> ()  [unwired: 2 in, 2 out]
              }
            }
          }
        }
        n632 = property on="Progress" class="Clust (strict)"("Visible"=FALSE) -> ()  [unwired: 2 in, 2 out]
      }
      event "Test Name": Mouse Enter {
        # "Populate the ring with the list of tests"
        n633 = event-data() -> ()  [unwired: 1 in, 1 out]
        n634 = call <vilib>:"NT Read String Array.vi"("Name"="TestMode/TestList") -> ("String Array"=w1045:string[])  [unwired: 9 in, 1 out]
        n635 = Build Array (concatenate)("Select the test to run...", w1045) -> (w1044:string[])
        n636 = property on="Test Name" class="Ring (strict)"("Strings []"=w1044) -> ()  [unwired: 2 in, 2 out]
      }
      event "Test Name": Value Change {
        w1047 = FALSE ("Visible")
        # "Tell the robot the test name to run"
        n637 = event-data() -> ("NewVal"=w1051:u16)  [unwired: 1 in]
        n638 = property on="Test Name" class="Ring (strict)"() -> ("Strings []"=w1052:string[])  [unwired: 2 in, 2 out]
        n639 = local write "Progress"(T6 {"Test Progress"=0, "Test Progress Text"=""} ("Progress")) -> ()
        n640 = Index Array(array=w1052, index=w1051) -> (element=w1050:string)
        n641 = call <vilib>:"NT Write String.vi"("String"=w1050, "Name"="TestMode/TestName") -> ()  [unwired: 9 in, 1 out]
        n642 = property on="Progress" class="Clust (strict)"("Visible"=TRUE) -> ()  [unwired: 2 in, 2 out]
        n643 = property on="Motor" class="Clust (strict)"("Visible"=w1047) -> ()  [unwired: 2 in, 2 out]
        n644 = property on="Test Slider" class="Slide (strict)"("Visible"=w1047) -> ()  [unwired: 2 in, 2 out]
        n645 = property on="On/Off" class="Bool (strict)"("Visible"=w1047) -> ()  [unwired: 2 in, 2 out]
        n646 = property on="Rev/Fwd" class="Clust (strict)"("Visible"=w1047) -> ()  [unwired: 2 in, 2 out]
        n647 = property on="Test Ring" class="Ring (strict)"("Visible"=w1047) -> ()  [unwired: 2 in, 2 out]
      }
      event "Select Auto": Mouse Enter {
        # "Populate the combo box with the list of autonomous options"
        n648 = event-data() -> ()  [unwired: 1 in, 1 out]
        n649 = call <vilib>:"NT Read String Array.vi"("Name"="Auto List") -> ("String Array"=w1054:string[])  [unwired: 9 in, 1 out]
        n650 = property on="Select Auto" class="CmbBox"("Strings[]"=w1054) -> ()  [unwired: 2 in, 2 out]
      }
      event "Select Auto": Value Change {
        # "User modified the Auto Selection. Write to NT variable so robot knows."
        n651 = event-data() -> ("NewVal"=w1057:string)  [unwired: 1 in]
        n652 = call <vilib>:"NT Write String.vi"("String"=w1057, "Name"="Auto Selector") -> ()  [unwired: 9 in, 1 out]
      }
      event "Command Selection": Value Change {
        # "Get the params and show in table"
        n653 = event-data() -> ("NewVal"=w1063:i32)  [unwired: 1 in]
        n654 = property on="Command Selection" class="MCListbox (strict)"() -> ("ItemNames"=w1061:string[][])  [unwired: 2 in, 2 out]
        n655 = call <vilib>:"WPI_DashboardUpdate Command Params.vi"("NewVal"=w1063, "Commands"=w1061, "Param Tbl"=w1062) -> ()  [unwired: 8 in, 1 out]
      }
      event "Execute Command": Value Change {
        # "Started one, Unique ID holds\nresponse"
        n656 = event-data() -> ()  [unwired: 1 in, 1 out]
        n657 = property on="Command Selection" class="MCListbox (strict)"() -> ("ItemNames"=w1074:string[][])  [unwired: 2 in, 2 out]
        n658 = Index Array(array=w1074, index (row)="Command Selection", index (col)=0) -> (element=w1072:string)
        n659 = call <vilib>:"Invoke Commands.vi"("Command Params"="Command Params", "Function Name"=w1072) -> ("Params"=w1068:u8, "Started"=w1067:bool)  [unwired: 7 in, 1 out]
        n660 = Array Subset(array="Command Params", length (row)=w1068) -> (w1069:string[][])  [unwired: 3 in]
        n661 = Select(t="Executing" ("Cmd Status"), s=w1067, f="" ("Cmd Status")) -> (s? t:f=→"Cmd Status":string)
      }
      event "Command Selection": Double Click {
        n662 = event-data() -> ("Row"=w1082:i32)  [unwired: 1 in]
        n663 = property on="Command Selection" class="MCListbox (strict)"() -> ("ItemNames"=w1085:string[][])  [unwired: 2 in, 2 out]
        n664 = local read "Command Params"() -> (w1081:string[][])
        n665 = Index Array(array=w1085, index (row)=w1082, index (col)=0) -> (element=w1083:string)
        n666 = call <vilib>:"Invoke Commands.vi"("Command Params"=w1081, "Function Name"=w1083) -> ("Params"=w1080:u8, "Started"=w1075:bool)  [unwired: 7 in, 1 out]
        n667 = Array Subset(array=w1081, length (row)=w1080) -> (w1079:string[][])  [unwired: 3 in]
        n668 = Select(t="Executing" ("Cmd Status"), s=w1075, f="" ("Cmd Status")) -> (s? t:f=w1076:string)
        n669 = local write "Cmd Status"(w1076) -> ()
      }
      event "CheckList": Double Click {
        # "Shift clears all"
        # "Update symbols on the listbox"
        n670 = event-data() -> ("PlatMods.Shift"=w1087:bool, "Row"=w1089:i32)  [unwired: 1 in]
        n671 = case shown="True" w1087 {
          tunnel: w1089 -> [w1093 _]
          tunnel: 1 -> [w1092 _]
          frame False {
            n672 = property on="CheckList" class="LstBox (strict)"() -> ("Item Symbols"=w1091:i32[])  [unwired: 2 in, 2 out]
            n673 = Replace Array Subset(array=w1091, new element=w1092, index=w1093) -> (w1090:i32[])
            n674 = property on="CheckList" class="LstBox (strict)"("Item Symbols"=w1090) -> ()  [unwired: 2 in, 2 out]
          }
          frame True {
            w1094 = 0 ("Top Row")
            n675 = property on="CheckList" class="LstBox (strict)"() -> ("Number of Rows"=w1096:u32)  [unwired: 2 in, 2 out]
            n676 = Initialize Array(0, w1096) -> (w1095:i32[])
            n677 = property on="CheckList" class="LstBox (strict)"("Top Row"=w1094, "Value"=w1094, "Item Symbols"=w1095) -> ()  [unwired: 2 in, 2 out]
          }
        }
      }
      event "CheckList": Key Down {
        # "Update symbols on the listbox\nLeft and right keys check and uncheck"
        n678 = event-data() -> ("VKey"=w1100:T22)  [unwired: 1 in]
        n679 = case shown="\"Left\", \"Right\"" w1100 {
          selector: w1100 -> [w1105 _]
          tunnel: eventvkey."Left" ("VKey") -> [w1103 _]
          frame "Left", "Right" {
            n680 = Equal?(x=w1103, y=w1105) -> (x = y?=w1104:bool)
            n681 = Select(t=0, s=w1104, f=1) -> (s? t:f=w1106:i32)
            n682 = property on="CheckList" class="LstBox (strict)"() -> ("Item Symbols"=w1109:i32[])  [unwired: 2 in, 2 out]
            n683 = Replace Array Subset(array=w1109, new element=w1106, index="CheckList") -> (w1108:i32[])
            n684 = property on="CheckList" class="LstBox (strict)"("Item Symbols"=w1108) -> ()  [unwired: 2 in, 2 out]
          }
          frame Default {
          }
        }
      }
      event "Motor.Enable": Value Change {
        # "When the test mode otor enable helper is set, update that\ntree row item's value"
        n685 = event-data() -> ("NewVal"=w1115:bool)  [unwired: 1 in]
        n686 = Unbundle("Motor") -> ("Value"=w1114:dbl)  [unwired: 1 out]
        n687 = Select(t=w1114, s=w1115, f=0.0) -> (s? t:f=w1112:dbl)
        n688 = call <vilib>:"NT Write Number.vi"("Numeric"=w1112, "Name"=w1111) -> ()  [unwired: 9 in, 1 out]
      }
      event "Test Slider": Value Change {
        # "When the test mode slider helper is set, update that\ntree row item's value"
        n689 = event-data() -> ("NewVal"=w1118:dbl)  [unwired: 1 in]
        n690 = call <vilib>:"NT Write Number.vi"("Numeric"=w1118, "Name"=w1119) -> ()  [unwired: 9 in, 1 out]
      }
      event "On/Off": Value Change {
        # "When the test mode on/off helper value is set, update that\ntree row item's value"
        n691 = event-data() -> ("NewVal"=w1123:bool)  [unwired: 1 in]
        n692 = Boolean To (0,1)(Boolean=w1123) -> (0, 1=w1122:i16)
        n693 = call <vilib>:"NT Write Number.vi"("Numeric"=w1122, "Name"=w1121) -> ()  [unwired: 9 in, 1 out]
      }
      event "Rev/Fwd": Value Change {
        # "When the test mode helper value for relays is set, update that\ntree row item's value"
        n694 = event-data() -> ("NewVal.Forward"=w1131:bool, "NewVal.Reverse"=w1130:bool)  [unwired: 1 in]
        n695 = Boolean To (0,1)(Boolean=w1131) -> (0, 1=w1127:i16)
        n696 = Boolean To (0,1)(Boolean=w1130) -> (0, 1=w1129:i16)
        n697 = Negate(x=w1129) -> (-x=w1128:i16)
        n698 = Add(x=w1127, y=w1128) -> (x+y=w1126:i16)
        n699 = call <vilib>:"NT Write Number.vi"("Numeric"=w1126, "Name"=w1125) -> ()  [unwired: 9 in, 1 out]
      }
      event "Test Ring": Value Change {
        # "When a test mode helper value is selected from the ring,\nset the tree item's variable to the string value"
        n700 = event-data() -> ("NewVal"=w1135:u16)  [unwired: 1 in]
        n701 = property on="Test Ring" class="Ring (strict)"() -> ("Strings []"=w1136:string[])  [unwired: 2 in, 2 out]
        n702 = Index Array(array=w1136, index=w1135) -> (element=w1134:string)
        n703 = call <vilib>:"NT Write String.vi"("String"=w1134, "Name"=w1133) -> ()  [unwired: 9 in, 1 out]
      }
      event "Rec Mode": Value Change {
        # "Update globals for recording mode and path to read log from.\nClear when logging and let NetworkTables set path for vision to\nuse."
        n704 = event-data() -> ("NewVal"=w1145:enum32{"Stop", "Record", "Playback"})  [unwired: 1 in]
        n705 = global write "WPI_DashboardLogging Global.vi" "Logging Filename"(path "") -> ()
        n706 = global write "WPI_DashboardLogging Global.vi" "Recording"(w1145) -> ()
        n707 = case shown="\"Playback\"" w1145 {
          tunnel: w1144 -> [_ w1147 w1156]
          tunnel: [_ _ w1155] -> w1142
          tunnel: [_ _ w1154] -> _
          tunnel: w1140 -> [_ _ w1152]
          tunnel: cluster{i32, i32} {-250, 170} -> [_ _ w1151]
          tunnel: [_ _ T23 {"Image Size"=TRUE, "Image Type"=TRUE, "Pixel Value"=TRUE, "ROI Information"=TRUE, "Zoom Factor"=FALSE} ("Image Information Shown:All Elements")] -> _
          tunnel: [_ _ TRUE ("Zoom Factor")] -> _
          tunnel: w1138 -> [_ _ w1148]
          frame Default {
          }
          frame "Stop", "Record" {
            # "Place Window too"
            n708 = invoke class="VI" method="FP.Close"(reference=w1147) -> (reference out=w1146:refnum<vi>)  [unwired: 2 in, 2 out]
            n709 = invoke class="VI" method="Abort VI"(reference=w1146) -> ()  [unwired: 2 in, 3 out]
          }
          frame "Playback" {
            n710 = call "Open Playback Panel.vi"("Offset"=w1151, "DB VI Ref"=w1152, "Playback in"=w1156) -> ("Playback out"=w1153:refnum<vi>)  [unwired: 8 in]
            n711 = register-events(w1153, w1148) -> (reference out=w1155:refnum<event-registration>, error out=w1154:errorcluster)  [unwired: 2 in]
          }
        }
        n712 = call <vilib>:"WPI_DashboardNT Log FieldName Cache.vi"("Operation"=enum16{"Lookup/Add", "Index", "Clear"}."Clear") -> ()  [unwired: 8 in, 3 out]
      }
      event Panel Close {
        w1158 = enum32{"Stop", "Record", "Playback"}."Stop" ("Rec Mode")
        # "Playback window has been closed, abort"
        n713 = event-data() -> ()  [unwired: 1 in, 4 out]
        n714 = local write "Rec Mode"(w1158) -> ()
        n715 = global write "WPI_DashboardLogging Global.vi" "Recording"(w1158) -> ()
      }
      event Panel Close {
        # "Abort playback window and ourself"
        n716 = event-data() -> ()  [unwired: 1 in, 4 out]
        n717 = invoke class="VI" method="FP.Close"(reference=w1162) -> (reference out=w1161:refnum<vi>)  [unwired: 2 in, 2 out]
        n718 = invoke class="VI" method="Abort VI"(reference=w1161) -> (error out=w1160:errorcluster)  [unwired: 2 in, 2 out]
        n719 = invoke class="VI" method="Abort VI"(error in=w1160) -> ()  [unwired: 2 in, 3 out]
      }
      event User Event {
        n720 = event-data() -> ("IDs"=w1169:cluster{"RPC field ID":u16, "Unique ID":u16}, "String"=w1168:string)  [unwired: 1 in]
        n721 = Bundle("IDs"=w1169, "String"=w1168) -> (w1167:T9)  [unwired: 1 in]
        n722 = call <vilib>:"Retrieve RPC Response.vi"("RPC Response"=w1167) -> ("Output"=w1165:string[][])  [unwired: 10 in]
        n723 = Build Array (concatenate)(w1163, w1165) -> (w1164:string[][])
        n724 = local write "Command Params"(w1164) -> ()
        n725 = local write "Cmd Status"("" ("Cmd Status")) -> ()
      }
      event "Tree": Double Click {
        n726 = event-data() -> ("PlatMods"=w1175:T26, "Tag"=w1172:string)  [unwired: 1 in]
        n727 = Unbundle(w1175) -> ("Shift"=w1174:bool)  [unwired: 4 out]
        n728 = String Subset(string=w1172, length (rest)=1 ("length (rest)")) -> (substring=w1171:string)  [unwired: 1 in]
        n729 = Not(x=w1174) -> (.not. x?=w1173:bool)
        n730 = case shown="\"/\"" w1171 {
          tunnel: w1172 -> [_ w1178]
          tunnel: w1173 -> [_ w1177]
          frame Default {
          }
          frame "/" {
            n731 = call <vilib>:"NT Update Persistence.vi"("Persistence"=w1177, "Name"=w1178) -> ()  [unwired: 9 in, 1 out]
          }
        }
      }
    }
  }
  n732 = local write "Dashboard Tab"(T1."Setup/Auto" ("Dashboard Tab")) -> ()
  n733 = property class="VI"() -> ("Panel"=w33:refnum<vi>)  [unwired: 2 in, 2 out]
  n734 = property class="Pnl"(reference=w33) -> ("Panes[]"=w34:refnum<vi>[])  [unwired: 1 in, 2 out]
  n735 = property on="On/Off" class="Bool (strict)"("Visible"=w20) -> ()  [unwired: 2 in, 2 out]
  n736 = property on="Motor" class="Clust (strict)"("Visible"=w20) -> ()  [unwired: 2 in, 2 out]
  n737 = property on="Progress" class="Clust (strict)"("Visible"=w20) -> ()  [unwired: 2 in, 2 out]
  n738 = property on="Test Ring" class="Ring (strict)"("Visible"=w20) -> ()  [unwired: 2 in, 2 out]
  n739 = property on="Rev/Fwd" class="Clust (strict)"("Visible"=w20) -> ()  [unwired: 2 in, 2 out]
  n740 = Index Array(array=w34) -> (element=w32:refnum<vi>)  [unwired: 1 in]
  n741 = while {
    tunnel: w32 -> [w1180]
    i -> [w1183]
    stop <- FALSE stop-if-true
    n742 = Wait (ms)(milliseconds to wait=u32 100) -> ()  [unwired: 1 out]
    n743 = case shown="\"Playback\"" "Rec Mode" {
      tunnel: w1183 -> [_ _ w1198]
      tunnel: [u32 2829099 ("Base Color") u32 11141120 ("Target Color") w1187] -> w1179
      frame "Stop", Default {
        # "Reset the color, extra updates don't cost much"
      }
      frame "Record" {
      }
      frame "Playback" {
        # "Playback"
        n744 = Quotient & Remainder(x=w1198, y=u32 50 ("milliseconds to wait")) -> (x-y*floor(x/y)=w1194:u32)  [unwired: 1 out]
        n745 = Divide(x=w1194, y=u32 50 ("milliseconds to wait")) -> (x/y=w1191:dbl)
        n746 = Multiply(x=6.283185307179586, y=w1191) -> (x*y=w1196:dbl)
        n747 = Sine(x=w1196) -> (sin(x)=w1195:dbl)
        n748 = Absolute Value(x=w1195) -> (abs(x)=w1188:dbl)
        n749 = call "Interpolate RGB Color.vi"("Proportion"=w1188, "Target Color"=u32 30976, "Base Color"=u32 2829099) -> ("Result Color"=w1187:u32)  [unwired: 8 in]
      }
    }
    n750 = property class="Pane"(reference=w1180, "PaneColor"=w1179) -> ()  [unwired: 1 in, 2 out]
  }
  n751 = while {
    tunnel: u16 1741 ("timeout ms (25000)") -> [w1200]
    stop <- FALSE stop-if-true
    n752 = TCP Create Listener(10:w1200) -> (0:w1199:errorcluster, 3:w1201:refnum<k5>)  [unwired: 4 in, 1 out]
    n753 = case shown="No Error" w1199 {
      selector: w1199 -> [w1203 _]
      tunnel: w1201 -> [w1204 _]
      frame No Error {
        n754 = while {
          tunnel: w1204 -> [w1207]
          tunnel: w1203 -> [w1206]
          stop <- FALSE stop-if-true
          n755 = TCP Wait On Listener(8:w1206, 11:w1207) -> (0:w1208:errorcluster, 4:w1209:refnum<k5>)  [unwired: 2 in, 3 out]
          n756 = local write "TCP"(w1209) -> ()
          n757 = case shown="No Error" w1208 {
            frame No Error {
            }
            frame Error {
              n758 = Wait (ms)(milliseconds to wait=u32 1000) -> ()  [unwired: 1 out]
            }
          }
        }
      }
      frame Error {
        n759 = Wait (ms)(milliseconds to wait=u32 1000) -> ()  [unwired: 1 out]
      }
    }
  }
  n760 = local write "Command Selection"(u16 0 ("milliseconds to wait")) -> ()
  n761 = local write "Command Params"(string[][] [] ("Command Params")) -> ()
  n762 = while {
    tunnel: w2 -> [_]
    stop <- FALSE stop-if-true
    # "Error Message Handling"
    n763 = property on="Actuator Testing" class="Ring (strict)"() -> ("RingText.Text"=w1243:string)  [unwired: 2 in, 2 out]
    n764 = local read "Master_Safety_Override_1"() -> (w1325:bool)
    n765 = local read "Master_Safety_Override_2"() -> (w1326:bool)
    n766 = local read "Drive_Train_Azimuth_Sensor"() -> (w1212:bool)
    n767 = local read "Arm_Calibrate_Joysticks"() -> (w1227:bool)
    n768 = local read "Turret_Azimuth_Failure"() -> (w1260:bool)
    n769 = Wait (ms)(milliseconds to wait=u32 200) -> ()  [unwired: 1 out]
    n770 = local read "Shooter_Motor_Failure"() -> (w1272:bool)
    n771 = local read "Drive_Train_Shifter"() -> (w1217:bool)
    n772 = local read "CAN_Bus_Fault"() -> (w1223:bool)
    n773 = local read "Drive_Train_Overheat"() -> (w1304:bool)
    n774 = local read "Arm_Calibrate_Turret"() -> (w1255:bool)
    n775 = Not Equal?(x=w1243, y="No_Test") -> (x != y?=w1250:bool)
    n776 = local read "Drive_Train_Azimuth"() -> (w1295:bool)
    n777 = call <vilib>:"Space Constant.vi"() -> ("String"=w1241:string)
    n778 = local read "Shooter_Overheat"() -> (w1280:bool)
    n779 = local read "Super_Test_Mode"() -> (w1314:bool)
    n780 = local read "Auto_Test_Mode"() -> (w1283:bool)
    n781 = local read "Intake_Overheat"() -> (w1264:bool)
    n782 = local read "Battery_Critical"() -> (w1311:bool)
    n783 = local read "Electrical_Fault"() -> (w1234:bool)
    n784 = local read "Out_Of_Range"() -> (w1268:bool)
    n785 = local read "Arm_Calibrate"() -> (w1291:bool)
    n786 = local read "Pressure_Leak"() -> (w1300:bool)
    n787 = local read "Arm_Climber"() -> (w1275:bool)
    n788 = Search and Replace String(input string=w1243, search string="_", replace string=w1241) -> (result string=w1244:string)  [unwired: 5 in, 3 out]
    n789 = local read "IMU_Failure"() -> (w1247:bool)
    n790 = local read "Match_End"() -> (w1238:bool)
    n791 = local read "Slow_Loop"() -> (w1307:bool)
    n792 = local read "Auto_Error"() -> (w1288:bool)
    n793 = Concatenate Strings("testing " ("string"), w1244) -> (w1253:string)
    n794 = And(x=w1325, y=w1326) -> (x .and. y?=w1316:bool)
    n795 = Bundle("swerve shifter failure, forced into low gear", "Drive_Train_Shifter"=w1217, 20.0) -> (w1216:cluster{string, "Drive_Train_Shifter":bool, dbl})  [unwired: 1 in]
    n796 = Bundle("swerve azimuth sensor failure", "Drive_Train_Azimuth_Sensor"=w1212, 20.0) -> (w1213:T27)  [unwired: 1 in]
    n797 = Bundle("safeties disengaged", w1316, 500.0) -> (w1320:cluster{string, bool, dbl})  [unwired: 1 in]
    n798 = Bundle("super test mode", "Super_Test_Mode"=w1314, 500.0) -> (w1319:cluster{string, "Super_Test_Mode":bool, dbl})  [unwired: 1 in]
    n799 = Bundle("battery low", "Battery_Critical"=w1311, 10.0) -> (w1318:cluster{string, "Battery_Critical":bool, dbl})  [unwired: 1 in]
    n800 = Bundle("control latency too high", "Slow_Loop"=w1307, 20.0) -> (w1308:cluster{string, "Slow_Loop":bool, dbl})  [unwired: 1 in]
    n801 = Bundle("drive train overheating", "Drive_Train_Overheat"=w1304, 10.0) -> (w1303:T28)  [unwired: 1 in]
    n802 = Bundle("pressure leak", "Pressure_Leak"=w1300, 10.0) -> (w1299:cluster{string, "Pressure_Leak":bool, dbl})  [unwired: 1 in]
    n803 = Bundle("swerve module failure and shutdown", "Drive_Train_Azimuth"=w1295, 20.0) -> (w1296:cluster{string, "Drive_Train_Azimuth":bool, dbl})  [unwired: 1 in]
    n804 = Bundle("ready to calibrate swerve modules", "Arm_Calibrate"=w1291, 60.0) -> (w1292:cluster{string, "Arm_Calibrate":bool, dbl})  [unwired: 1 in]
    n805 = Bundle("autonomous play failure", "Auto_Error"=w1288, 20.0) -> (w1287:cluster{string, "Auto_Error":bool, dbl})  [unwired: 1 in]
    n806 = Bundle("autonomous test mode", "Auto_Test_Mode"=w1283, 500.0) -> (w1284:cluster{string, "Auto_Test_Mode":bool, dbl})  [unwired: 1 in]
    n807 = Bundle("shooter overheating", "Shooter_Overheat"=w1280, 10.0) -> (w1279:cluster{string, "Shooter_Overheat":bool, dbl})  [unwired: 1 in]
    n808 = Bundle("climber is armed", "Arm_Climber"=w1275, 30.0) -> (w1276:cluster{string, "Arm_Climber":bool, dbl})  [unwired: 1 in]
    n809 = Bundle("shooter motor failure", "Shooter_Motor_Failure"=w1272, 10.0) -> (w1271:T29)  [unwired: 1 in]
    n810 = Bundle("out of range", "Out_Of_Range"=w1268, 5.0) -> (w1267:cluster{string, "Out_Of_Range":bool, dbl})  [unwired: 1 in]
    n811 = Bundle("intake overheating", "Intake_Overheat"=w1264, 10.0) -> (w1263:cluster{string, "Intake_Overheat":bool, dbl})  [unwired: 1 in]
    n812 = Bundle("turret azimuth failure, turret disabled", "Turret_Azimuth_Failure"=w1260, 20.0) -> (w1259:T30)  [unwired: 1 in]
    n813 = Bundle("ready to calibrate turret", "Arm_Calibrate_Turret"=w1255, 60.0) -> (w1256:T31)  [unwired: 1 in]
    n814 = Bundle(w1253, w1250, 500.0) -> (w1249:cluster{string, bool, dbl})  [unwired: 1 in]
    n815 = Bundle("IMU failure, auto targeting disabled", "IMU_Failure"=w1247, 20.0) -> (w1245:cluster{string, "IMU_Failure":bool, dbl})  [unwired: 1 in]
    n816 = Bundle("let's blow this thing and go home", "Match_End"=w1238, 1000.0) -> (w1237:cluster{string, "Match_End":bool, dbl})  [unwired: 1 in]
    n817 = Bundle("electrical bus fault, power down immediately", "Electrical_Fault"=w1234, 10.0) -> (w1233:cluster{string, "Electrical_Fault":bool, dbl})  [unwired: 1 in]
    n818 = Bundle("ready to calibrate joysticks, wait ten seconds after pressing calibrate", "Arm_Calibrate_Joysticks"=w1227, 60.0) -> (w1228:T32)  [unwired: 1 in]
    n819 = Bundle("CAN bus fault, check wiring", "CAN_Bus_Fault"=w1223, 20.0) -> (w1225:cluster{string, "CAN_Bus_Fault":bool, dbl})  [unwired: 1 in]
    n820 = local read "Audible_Warnings_Enabled"() -> (w1226:bool)
    n821 = Build Array(w1320, w1319, w1318, w1308, w1303, w1299, w1296, w1292, w1287, w1284, w1279, w1276, w1271, w1267, w1263, w1259, w1256, w1249, w1245, w1237, w1233, w1228, w1225, w1216, w1213) -> (w1317:T33)
    n822 = call "ErrorMessageBuilder.vi"("Errors"=w1317) -> ("Combined Error String"=w1220:string)
    n823 = call <vilib>:"Connection Info.vi"() -> ("Connected"=w1231:bool)  [unwired: 10 in, 1 out]
    n824 = Not Equal?(x="", y=w1220) -> (x != y?=w1221:bool)
    n825 = Compound Arithmetic op=AND(w1226, w1231, w1221) -> (w1232:bool)
    n826 = case shown="True" w1232 {
      tunnel: w1220 -> [_ w1330]
      frame False {
      }
      frame True {
        n827 = call "TextToSpeech.vi"("Text To Be Spoken"=w1330) -> ()  [unwired: 9 in, 2 out]
      }
    }
    n828 = case shown="True" w1221 {
      tunnel: w1220 -> [_ w1329]
      frame False {
      }
      frame True {
        "Combined Error String" <- w1329
      }
    }
  }
  n829 = global write "WPI_DashboardLogging Global.vi" "Recording"(w26) -> ()
  n830 = local write "Rec Mode"(w26) -> ()
  n831 = call <vilib>:"NT Write String.vi"("String"="Select Auto", "Name"="Auto Selector") -> ()  [unwired: 9 in, 1 out]
  n832 = while {
    stop <- FALSE stop-if-true
    # "Set window properties"
    n833 = Not(x="Dock_Dashboard") -> (.not. x?=w1331:bool)
    n834 = First Call?() -> (First Call?: T/F=w1336:bool)
    n835 = Wait (ms)(milliseconds to wait=u32 10) -> ()  [unwired: 1 out]
    n836 = Compound Arithmetic op=OR(w1331, w1336) -> (w1333:bool)
    n837 = control-ref of="This VI"() -> (w1334:refnum<vi>)
    n838 = call "EdgeTrigger.vi"("Input Signal"=w1333) -> ("Falling Edge Trigger"=w1332:bool)  [unwired: 2 out]
    n839 = case shown="True" w1333 {
      tunnel: w1334 -> [w1341 w1348]
      tunnel: w1332 -> [w1339 _]
      frame False {
        n840 = case shown="True" w1339 {
          tunnel: T34 {"Left"=100, "Top"=100, "Right"=1390, "Bottom"=585} ("Front Panel Window:Window Bounds") -> [_ w1347]
          tunnel: w1341 -> [w1344 w1346]
          tunnel: [w1344 w1345] -> w1340
          frame False {
          }
          frame True {
            n841 = property class="VI"(reference=w1346, "Front Panel.WinBounds"=w1347) -> (reference out=w1345:refnum<vi>)  [unwired: 1 in, 1 out]
          }
        }
        n842 = property class="VI"(reference=w1340, "Front Panel.TitleBarVis"=TRUE ("Front Panel Window:Title Bar Visible")) -> ()  [unwired: 1 in, 2 out]
      }
      frame True {
        n843 = property class="VI"(reference=w1348, "Front Panel.WinBounds"=T34 {"Left"=0, "Top"=0, "Right"=1290, "Bottom"=485} ("Front Panel Window:Window Bounds"), "Front Panel.TitleBarVis"=FALSE ("Front Panel Window:Title Bar Visible")) -> ()  [unwired: 1 in, 2 out]
      }
    }
  }
